vi "cursor window logic V2.vi"(4 "h. offset":dbl, 6 "CursIdx":i32, 7 "cursor window action":T2=enum."check", 8 "window":dbl=nan, 9 "center":dbl=nan, 10 "cursor window in":refnum<vi>, 11 "cursor window init":T1={"left"=2378.60310421286, "right "=2421.6740576496672, "center"=2421.6740576496672, "window"=2421.6740576496672, "cursors"=[], "relative"=0, "absolute"=0, "fixed vertical offset"=2421.6740576496672, "vertical offset"=2421.6740576496672, "skew"=2421.6740576496672, "default window frac"=2421.6740576496672, "kind"=enum."skewed", "skew.left"=2421.6740576496672, "skew.right"=2421.6740576496672, "Plot ref"=refnum, "wing order"=enum."back"}) -> (2 "cursor window out":refnum<vi>, 3 "cursor window out":T1={"left"=2378.60310421286, "right "=2421.6740576496672, "center"=2421.6740576496672, "window"=2421.6740576496672, "cursors"=[], "relative"=0, "absolute"=0, "fixed vertical offset"=2421.6740576496672, "vertical offset"=2421.6740576496672, "skew"=2421.6740576496672, "default window frac"=2421.6740576496672, "kind"=enum."skewed", "skew.left"=2421.6740576496672, "skew.right"=2421.6740576496672, "Plot ref"=refnum, "wing order"=enum."back"})   [LabVIEW 2015]
uses:
  cursor window action.ctl
  cursor winow.ctl
  stack action -- control.ctl
  Q - not nan -- real.vi
  Q - not nan -- integer.vi
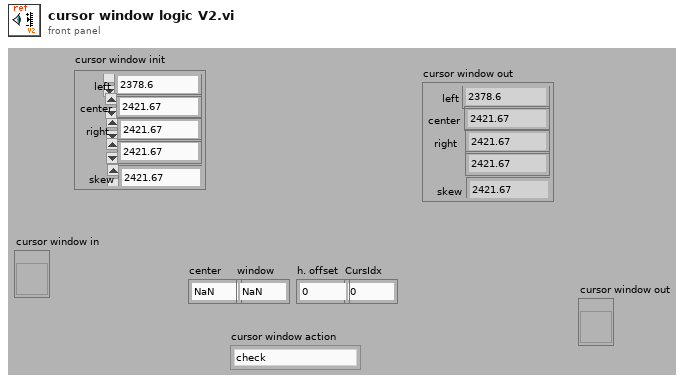
[diagram p1: front panel]
types:
  T1 = typedef "cursor winow.ctl" = cluster{"left":dbl, "right ":dbl, "center":dbl, "window":dbl, "cursors":i32[], "relative":i32, "absolute":i32, "fixed vertical offset":dbl, "vertical offset":dbl, "skew":dbl, "default window frac":dbl, "kind":enum16{"symmetric", "skewed", "fancy"}, "skew.left":dbl, "skew.right":dbl, "Plot ref":refnum<vi>, "wing order":enum16{"forw", "back"}}
  T2 = typedef "cursor window action.ctl" = enum16{"balance", "h. offset change", "cursor moves", "change center", "change window", "init", "check", "reset", "set y to middle", "idle", "-write all Y", "-write left.X", "-write center.X", "-write right.X", "-write all X", "-change center", "-change window", "-change skew", "-read cursor 2", "-read cursor 1", "-read cursor 0", "-read all cursors", "-reset", "-read plot scale", "-set y to middle", "-Q: center.Y is visible", "-Q: window is visible", "-parse center.Y", "-right left from center", "-left move", "-right move", "-set center.Y", "-empty", "-set cursors to default", "-check", "-write center.Y", "-copy cursor 1", "-copy cursor 0", "-copy cursor 2", "move right", "move left", "shrink", "broaden", "skew up", "skew down", "-write plot scale", "zoom X", "change cen&win", "zoom to all data"}
  T3 = typedef "stack action -- control.ctl" = enum16{"push", "pop", "check", "init"}
  T4 = cluster{"center":dbl, "window":dbl, "h.offset":dbl, "cursor window":T1}
  T5 = cluster{"right.Y":dbl, "right.X":dbl, "left.X":dbl, "left.Y":dbl, "center.X":dbl, "center.Y":dbl, "scale.x.max":dbl, "scale.x.min":dbl, "scale.y.range":dbl, "scale.y.min":dbl, "scale.x.range":dbl, "scale.y.max":dbl, "skew":dbl, "cursor":i32, "scale.x.center":dbl, "scale.x.halfwidth":dbl, "scale.y.center":dbl, "scale.y.halfwidth":dbl}
  T6 = cluster{"left":dbl, "right ":dbl, "center":dbl, "window":dbl, "cursors":i32[], "relative":i32, "absolute":i32, "fixed vertical offset":dbl, "vertical offset":dbl, "skew":dbl, "default window frac":dbl, "kind":enum16{"symmetric", "skewed", "fancy"}, "skew.left":dbl, "skew.right":dbl, "Plot ref":refnum<vi>, "wing order":enum16{"forw", "back"}}
  T7 = typedef "comparison control.ctl" = enum16{"not a number", "above", "in range", "below"}
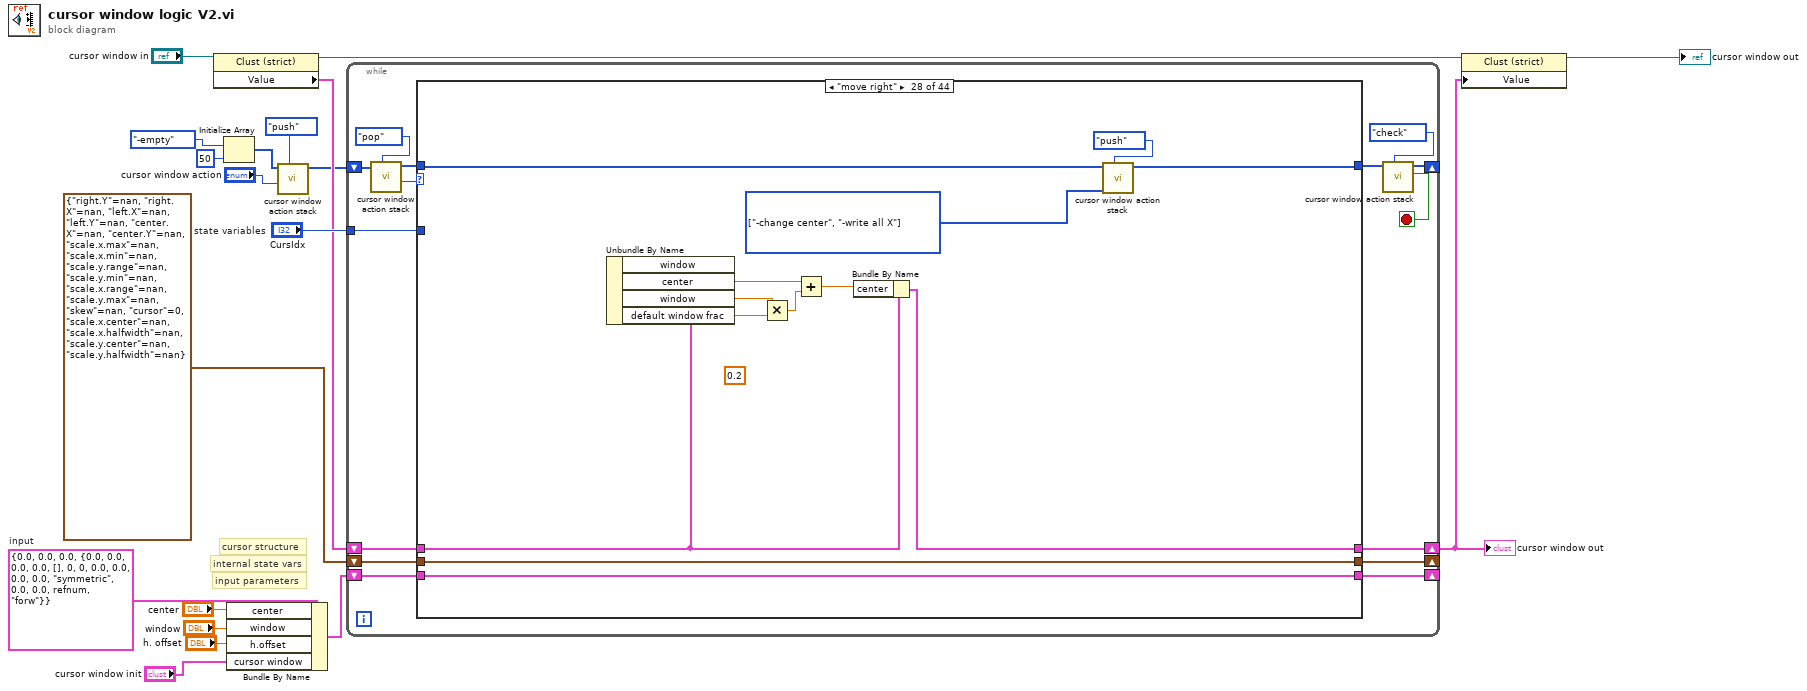
[diagram p0: block diagram]
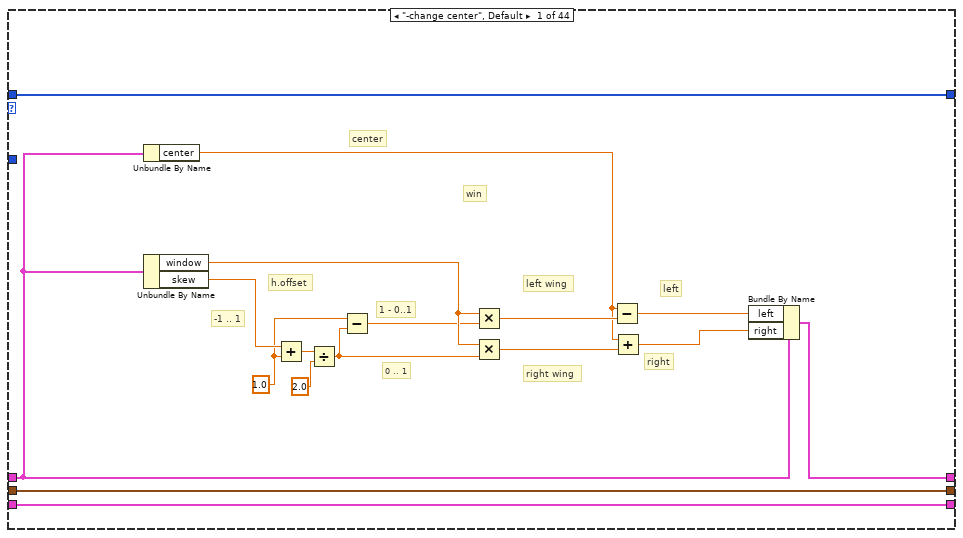
[diagram p2: hidden frame]
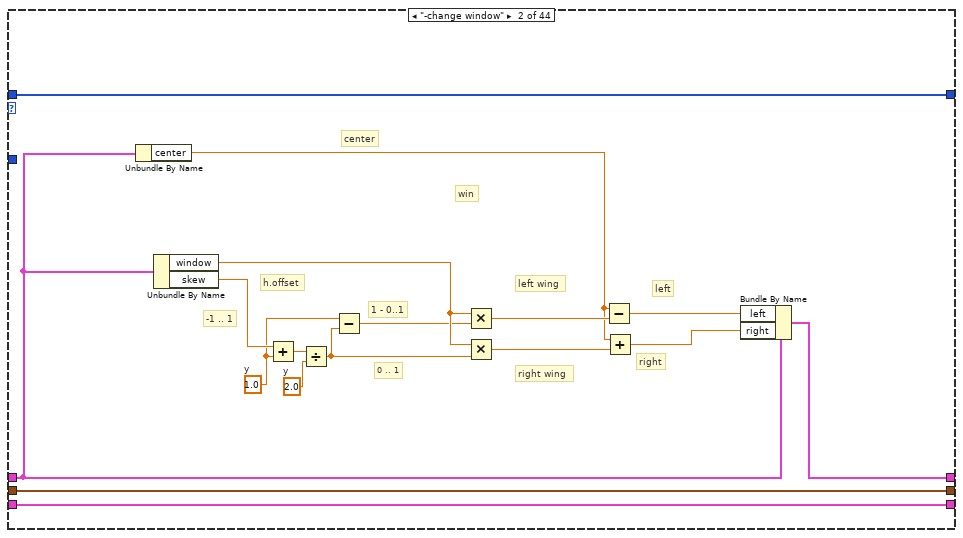
[diagram p3: hidden frame]
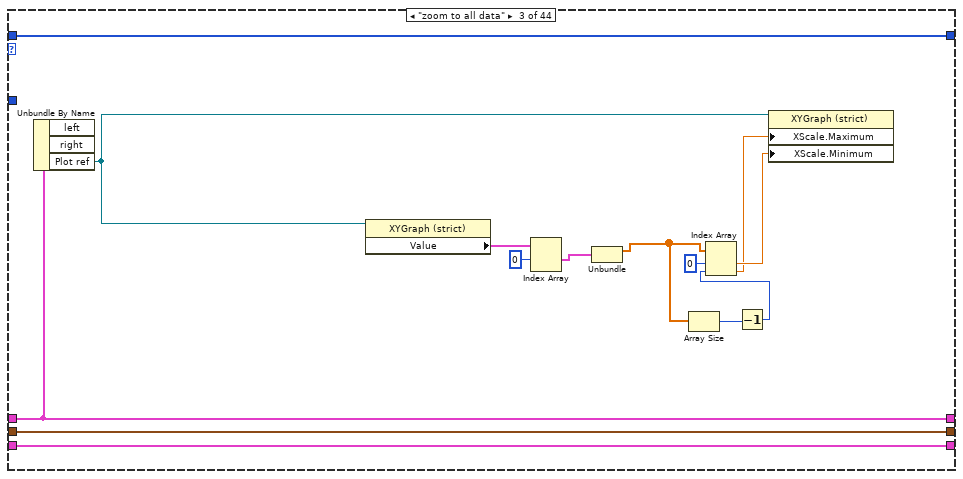
[diagram p4: hidden frame]
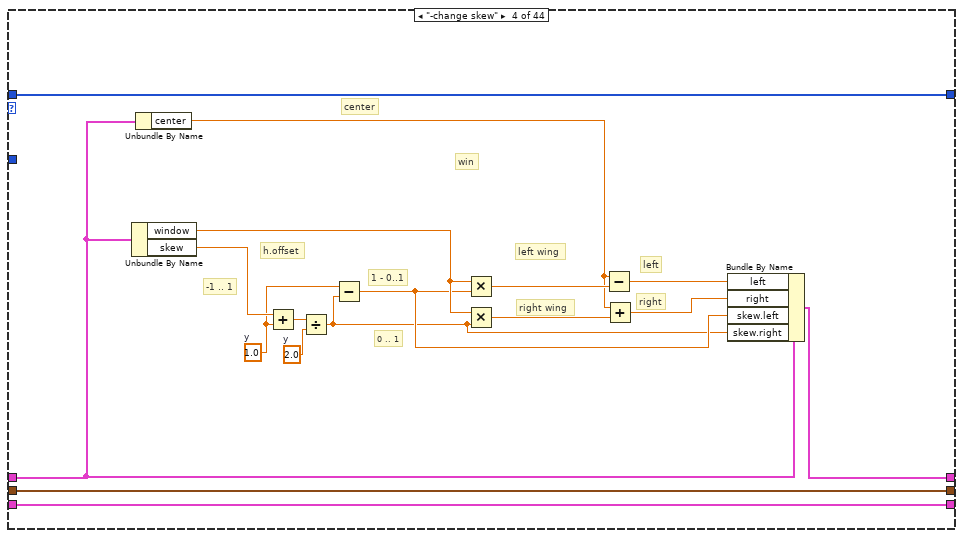
[diagram p5: hidden frame]
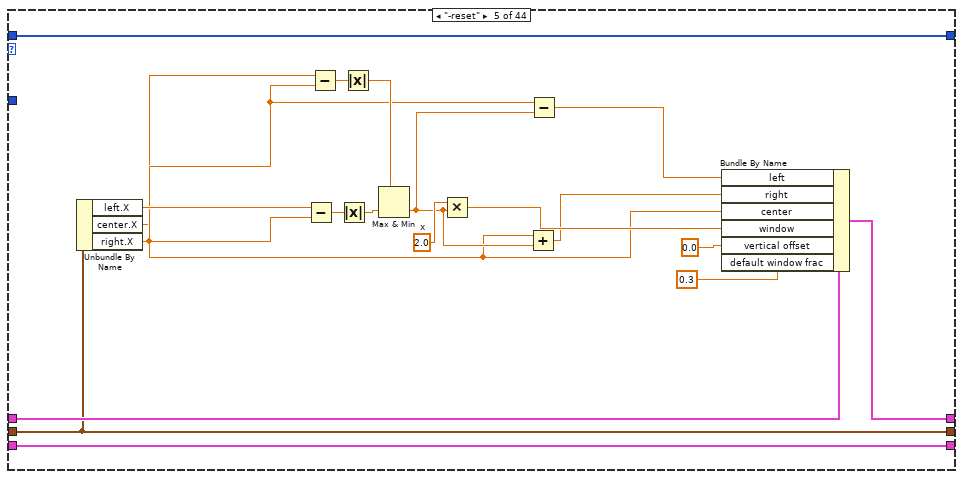
[diagram p6: hidden frame]
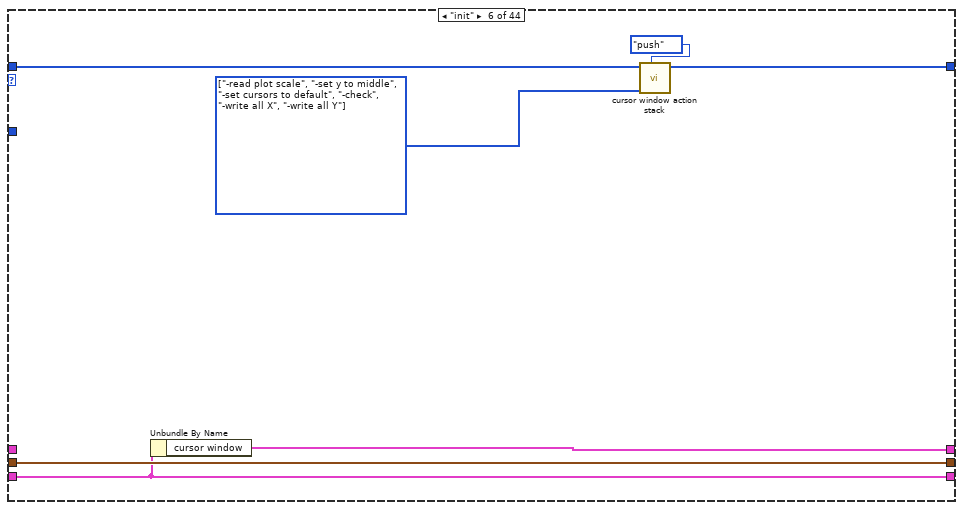
[diagram p7: hidden frame]
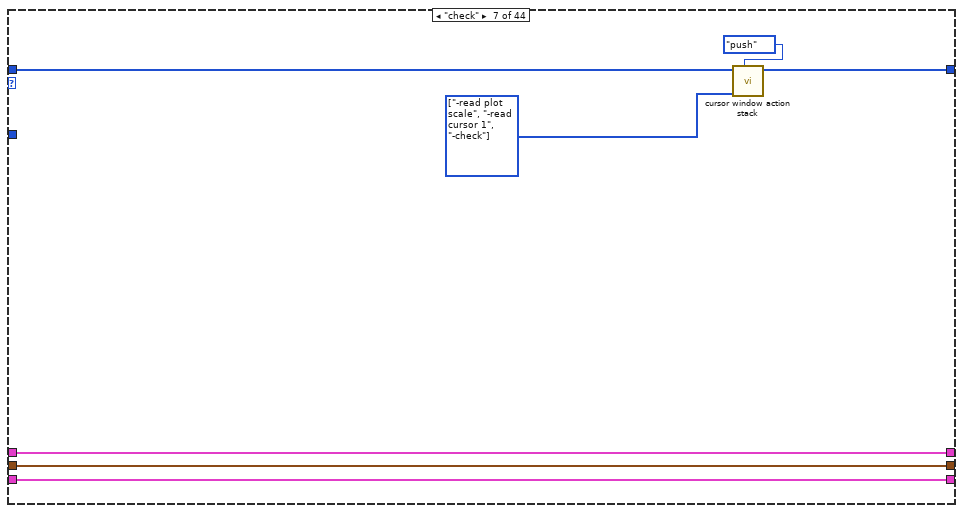
[diagram p8: hidden frame]
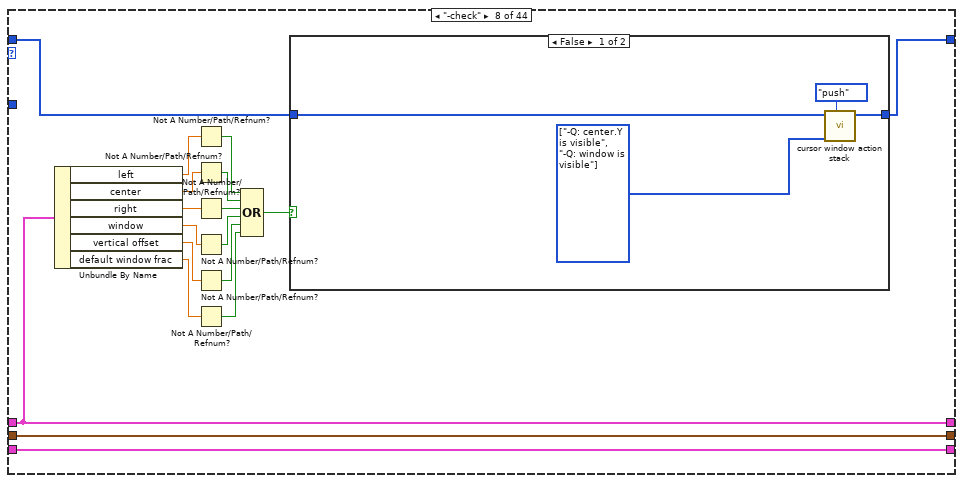
[diagram p9: hidden frame]
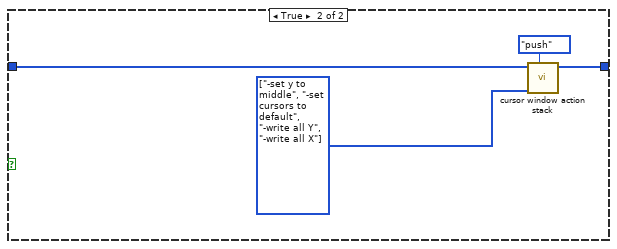
[diagram p10: hidden frame]
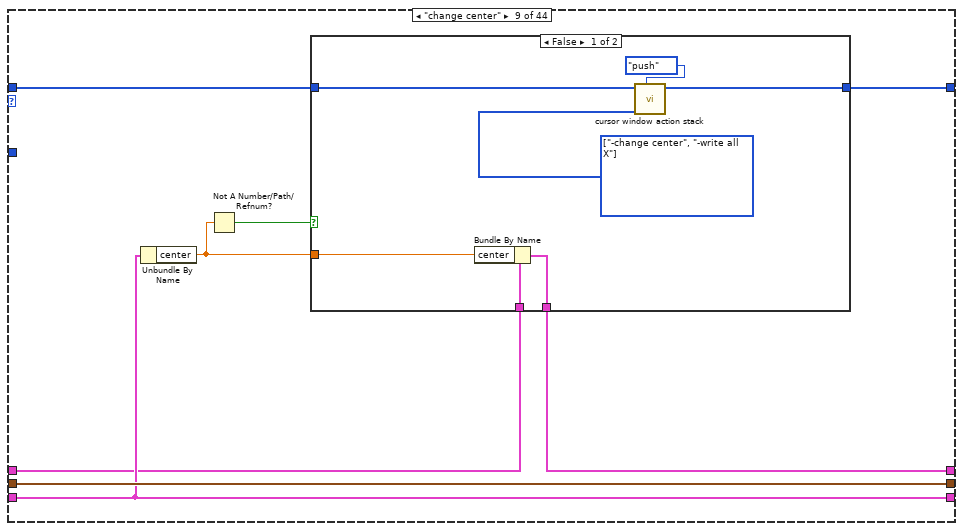
[diagram p11: hidden frame]
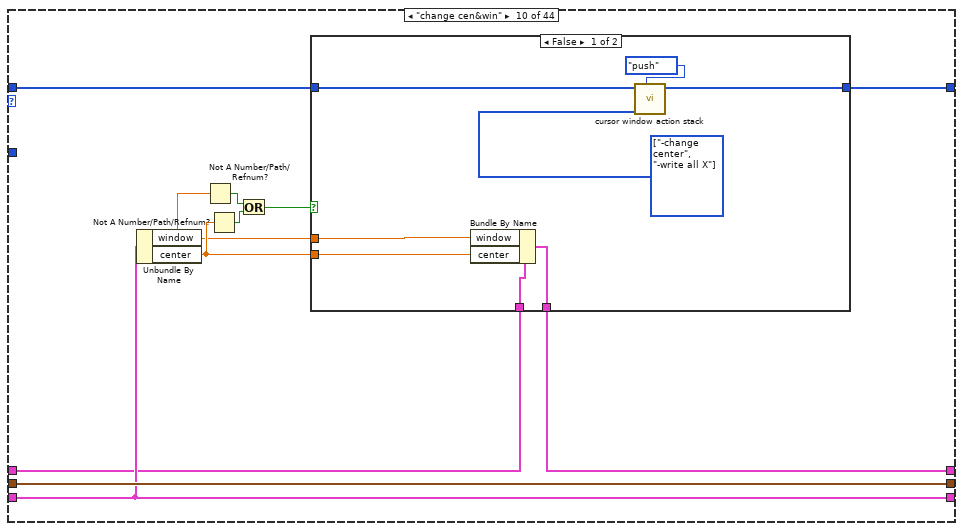
[diagram p13: hidden frame]
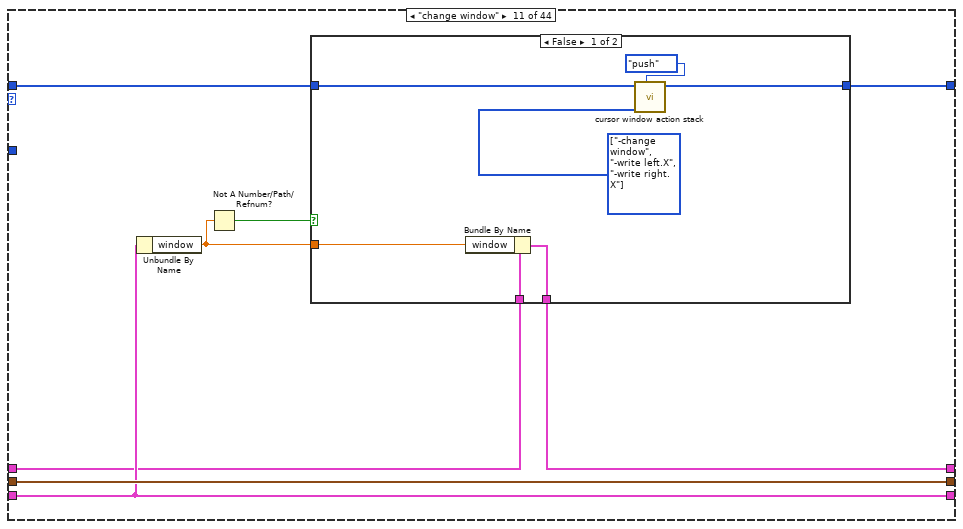
[diagram p15: hidden frame]
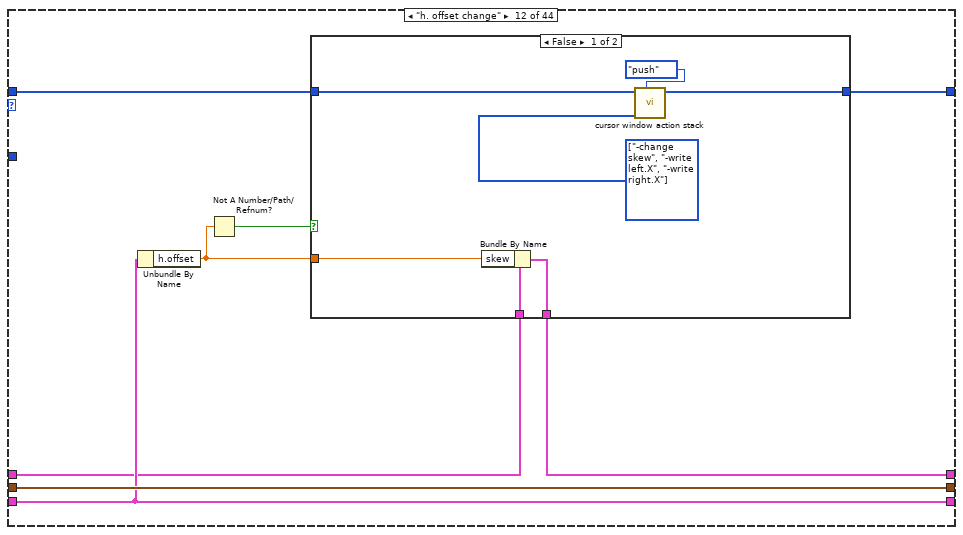
[diagram p17: hidden frame]
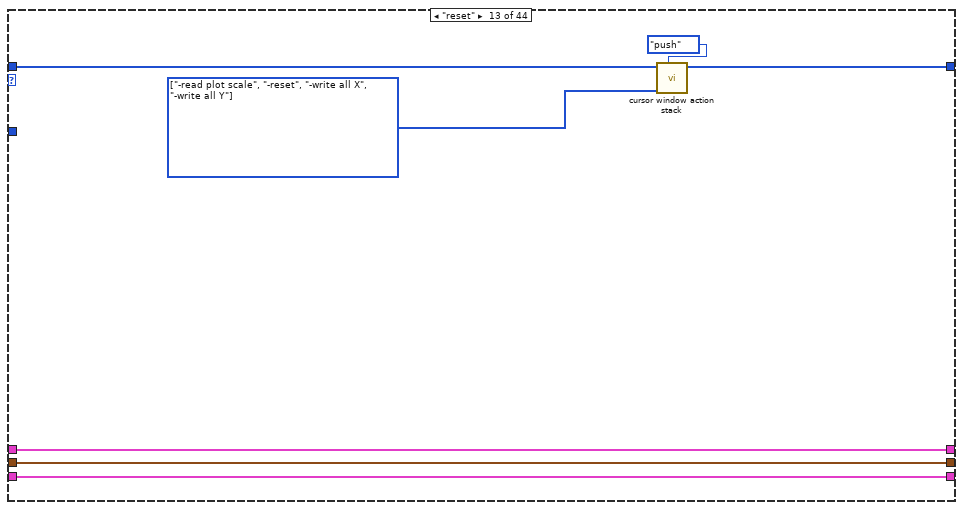
[diagram p19: hidden frame]
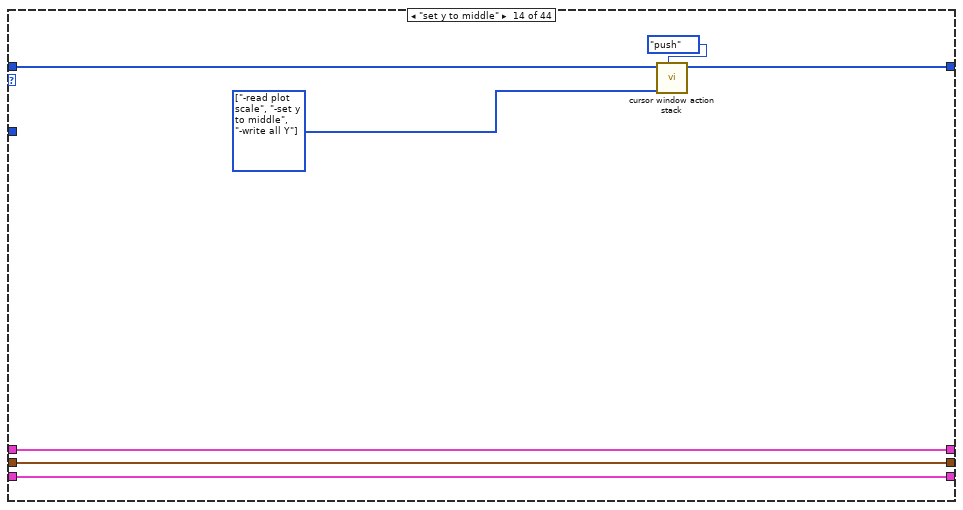
[diagram p20: hidden frame]
diagram:
  w17 = T4 {"center"=0.0, "window"=0.0, "h.offset"=0.0, "cursor window"={"left"=0.0, "right "=0.0, "center"=0.0, "window"=0.0, "cursors"=[], "relative"=0, "absolute"=0, "fixed vertical offset"=0.0, "vertical offset"=0.0, "skew"=0.0, "default window frac"=0.0, "kind"=enum."symmetric", "skew.left"=0.0, "skew.right"=0.0, "Plot ref"=refnum, "wing order"=enum."forw"}}  # input
  w18 = T5 {"right.Y"=nan, "right.X"=nan, "left.X"=nan, "left.Y"=nan, "center.X"=nan, "center.Y"=nan, "scale.x.max"=nan, "scale.x.min"=nan, "scale.y.range"=nan, "scale.y.min"=nan, "scale.x.range"=nan, "scale.y.max"=nan, "skew"=nan, "cursor"=0, "scale.x.center"=nan, "scale.x.halfwidth"=nan, "scale.y.center"=nan, "scale.y.halfwidth"=nan}  # state variables
  # "input parameters"
  # "internal state vars"
  # "cursor structure"
  n1 = property class="Clust (strict)"(reference="cursor window in") -> (reference out=w19:refnum<vi>, "Value"=w11:T6)  [unwired: 1 in, 1 out]
  n2 = Initialize Array(cursor_window_action."-empty" ("cursor window action"), 50 ("dimension size")) -> (w4:T2[])
  n3 = Bundle By Name(cluster=w17, "center"="center", "window"="window", "h.offset"="h. offset", "cursor window"="cursor window init") -> (w13:T4)
  n4 = call "cursor window action stack.vi"("stack action"=stack_action_--_control."push", "cursor window action"="cursor window action", "command stack"=w4) -> ("command stack out"=w3:T2[])  [unwired: 6 in, 2 out]
  n5 = while {
    shift-right: [w27] -> _
    shift-left: w3 -> [w33]
    shift-right: [w20] -> w10
    shift-left: w11 -> [w34]
    shift-right: [w24] -> _
    shift-left: w13 -> [w25]
    shift-right: [w22] -> _
    shift-left: w18 -> [w23]
    tunnel: "CursIdx" -> [w21]
    stop <- w26 stop-if-true
    n6 = call "cursor window action stack.vi"("stack action"=stack_action_--_control."pop", "command stack"=w33) -> ("cursor window action out"=w32:T2, "command stack out"=w30:T2[])  [unwired: 7 in, 1 out]
    n7 = case shown="\"move right\"" w32 {
      tunnel: w34 -> [w36 w53 w79 w86 w108 _ w126 w136 w160 w181 w198 w215 w231 w238 w255 w289 w324 w363 w395 w406 w413 w432 w439 w468 w481 w489 w513 w519 w539 w545 w558 w579 w618 w652 w692 w714 w728 w745 w764 w777 w786 w809 w822 w836]
      tunnel: [w40 w57 w82 w90 w107 w120 w129 w133 w165 w185 w203 w220 w234 w241 w252 w286 w326 w364 w396 w404 w422 w438 w455 w470 w483 w487 w514 w527 w540 w554 w562 w583 w616 w654 w709 w727 w742 w759 w773 w785 w807 w821 w835 w849] -> w28
      tunnel: w30 -> [w40 w57 w82 w90 w107 w121 w130 w134 w164 w184 w202 w219 w235 w242 w252 w286 w326 w351 w396 w404 w422 w438 w455 w470 w483 w488 w515 w528 w541 w555 w563 w584 w616 w655 w709 w727 w742 w759 w773 w785 w807 w821 w835 w849]
      tunnel: w25 -> [w37 w54 w80 w87 w106 w124 w127 w137 w163 w183 w201 w218 w237 w244 w254 w288 w325 w356 w393 w407 w421 w437 w458 w471 w484 w495 w509 w525 w535 w552 w559 w580 w634 w659 w694 w716 w734 w752 w766 w779 w788 w811 w825 w839]
      tunnel: [w37 w54 w80 w87 w106 w124 w127 w137 w163 w183 w201 w218 w237 w244 w254 w288 w325 w356 w393 w407 w421 w437 w458 w471 w484 w495 w509 w525 w535 w552 w559 w580 w634 w659 w694 w716 w734 w752 w766 w779 w788 w811 w825 w839] -> w24
      tunnel: w23 -> [w39 w56 w81 w89 w105 w125 w128 w138 w166 w186 w204 w221 w236 w243 w253 w287 w330 w357 w394 w409 w418 w436 w457 w462 w475 w491 w510 w526 w536 w553 w560 w581 w622 w658 w695 w713 w735 w753 w767 w776 w796 w815 w829 w843]
      tunnel: [w39 w56 w81 w89 w105 w125 w128 w138 w166 w186 w204 w221 w236 w243 w253 w287 w329 w357 w394 w409 w417 w436 w456 w462 w475 w490 w510 w526 w536 w553 w560 w581 w625 w658 w695 w713 w735 w753 w767 w776 w795 w814 w828 w842] -> w22
      tunnel: w21 -> [_ _ _ _ _ _ _ _ _ _ _ _ _ _ _ _ _ w354 _ _ _ _ _ _ _ _ _ _ _ _ _ _ _ _ _ _ _ _ _ _ _ _ _ _]
      tunnel: [w35 w52 w79 w85 w101 w119 w126 w136 w159 w180 w197 w214 w231 w238 w245 w279 w324 w355 w395 w405 w412 w428 w439 w468 w481 w489 w512 w518 w538 w544 w561 w582 w614 w651 w692 w714 w728 w745 w764 w777 w786 w809 w822 w836] -> w20
      frame "-change center", Default {
        w45 = 1.0 ("y")
        # "1 - 0..1"
        # "right"
        # "left"
        # "win"
        # "h.offset"
        # "center"
        # "left wing"
        # "right wing"
        # "0 .. 1"
        # "-1 .. 1"
        n8 = Unbundle By Name(w36) -> ("center"=w38:dbl)
        n9 = Unbundle By Name(w36) -> ("window"=w50:dbl, "skew"=w51:dbl)
        n10 = Add(x=w51, y=w45) -> (x+y=w46:dbl)
        n11 = Divide(x=w46, y=2.0) -> (x/y=w42:dbl)
        n12 = Subtract(x=w45, y=w42) -> (x-y=w41:dbl)
        n13 = Multiply(x=w50, y=w41) -> (x*y=w44:dbl)
        n14 = Multiply(x=w50, y=w42) -> (x*y=w43:dbl)
        n15 = Subtract(x=w38, y=w44) -> (x-y=w49:dbl)
        n16 = Add(x=w38, y=w43) -> (x+y=w48:dbl)
        n17 = Bundle By Name(cluster=w36, "left"=w49, "right"=w48) -> (w35:T1)
      }
      frame "-change window" {
        w62 = 1.0  # y
        w64 = 2.0  # y
        # "1 - 0..1"
        # "right"
        # "left"
        # "win"
        # "h.offset"
        # "center"
        # "left wing"
        # "right wing"
        # "0 .. 1"
        # "-1 .. 1"
        n18 = Unbundle By Name(w53) -> ("center"=w55:dbl)
        n19 = Unbundle By Name(w53) -> ("window"=w67:dbl, "skew"=w68:dbl)
        n20 = Add(x=w68, y=w62) -> (x+y=w63:dbl)
        n21 = Divide(x=w63, y=w64) -> (x/y=w59:dbl)
        n22 = Subtract(x=w62, y=w59) -> (x-y=w58:dbl)
        n23 = Multiply(x=w67, y=w58) -> (x*y=w61:dbl)
        n24 = Multiply(x=w67, y=w59) -> (x*y=w60:dbl)
        n25 = Subtract(x=w55, y=w61) -> (x-y=w66:dbl)
        n26 = Add(x=w55, y=w60) -> (x+y=w65:dbl)
        n27 = Bundle By Name(cluster=w53, "left"=w66, "right"=w65) -> (w52:T1)
      }
      frame "zoom to all data" {
        n28 = Unbundle By Name(w79) -> ("Plot ref"=w78:refnum<vi>)  [unwired: 2 out]
        n29 = property class="XYGraph (strict)"(reference=w78) -> ("Value"=w77:cluster{"all rows":dbl[], "all rows":dbl[]}[])  [unwired: 1 in, 2 out]
        n30 = Index Array(array=w77, index #1=0 ("index")) -> (element #1=w75:cluster{"all rows":dbl[], "all rows":dbl[]})  [unwired: 1 in, 1 out]
        n31 = Unbundle(w75) -> ("all rows"=w73:dbl[])  [unwired: 1 out]
        n32 = Array Size(array=w73) -> (size(s)=w72:i32)
        n33 = Decrement(x=w72) -> (x-1=w71:i32)
        n34 = Index Array(array=w73, index #1=0 ("index"), index #2=w71) -> (element #1=w70:dbl, element #2=w69:dbl)
        n35 = property class="XYGraph (strict)"(reference=w78, "XScale.Maximum"=w69, "XScale.Minimum"=w70) -> ()  [unwired: 1 in, 2 out]
      }
      frame "-change skew" {
        w93 = 1.0  # y
        w95 = 2.0  # y
        # "1 - 0..1"
        # "right"
        # "left"
        # "win"
        # "h.offset"
        # "center"
        # "left wing"
        # "right wing"
        # "0 .. 1"
        # "-1 .. 1"
        n36 = Unbundle By Name(w86) -> ("window"=w98:dbl, "skew"=w99:dbl)
        n37 = Unbundle By Name(w86) -> ("center"=w88:dbl)
        n38 = Add(x=w99, y=w93) -> (x+y=w94:dbl)
        n39 = Divide(x=w94, y=w95) -> (x/y=w83:dbl)
        n40 = Subtract(x=w93, y=w83) -> (x-y=w84:dbl)
        n41 = Multiply(x=w98, y=w84) -> (x*y=w92:dbl)
        n42 = Multiply(x=w98, y=w83) -> (x*y=w91:dbl)
        n43 = Subtract(x=w88, y=w92) -> (x-y=w97:dbl)
        n44 = Add(x=w88, y=w91) -> (x+y=w96:dbl)
        n45 = Bundle By Name(cluster=w86, "left"=w97, "right"=w96, "skew.left"=w84, "skew.right"=w83) -> (w85:T1)
      }
      frame "-reset" {
        w114 = 2.0  # x
        n46 = Unbundle By Name(w105) -> ("left.X"=w104:dbl, "center.X"=w102:dbl, "right.X"=w103:dbl)
        n47 = Subtract(x=w104, y=w103) -> (x-y=w117:dbl)
        n48 = Subtract(x=w102, y=w103) -> (x-y=w118:dbl)
        n49 = Absolute Value(x=w117) -> (abs(x)=w115:dbl)
        n50 = Absolute Value(x=w118) -> (abs(x)=w116:dbl)
        n51 = Max & Min(x=w116, y=w115) -> (min(x,y)=w112:dbl)  [unwired: 1 out]
        n52 = Multiply(x=w114, y=w112) -> (x*y=w113:dbl)
        n53 = Add(x=w103, y=w112) -> (x+y=w110:dbl)
        n54 = Subtract(x=w103, y=w112) -> (x-y=w111:dbl)
        n55 = Bundle By Name(cluster=w108, "left"=w111, "right"=w110, "center"=w103, "window"=w113, "vertical offset"=0.0, "default window frac"=0.3) -> (w101:T1)
      }
      frame "init" {
        w122 = T2[] [enum."-read plot scale", enum."-set y to middle", enum."-set cursors to default", enum."-check", enum."-write all X", enum."-write all Y"] items=["balance", "h. offset change", "cursor moves", "change center", "change window", "init", "check", "reset", "set y to middle", "idle", "-write all Y", "-write left.X", "-write center.X", "-write right.X", "-write all X", "-change center", "-change window", "-change skew", "-read cursor 2", "-read cursor 1", "-read cursor 0", "-read all cursors", "-reset", "-read plot scale", "-set y to middle", "-Q: center.Y is visible", "-Q: window is visible", "-parse center.Y", "-right left from center", "-left move", "-right move", "-set center.Y", "-empty", "-set cursors to default", "-check", "-write center.Y", "-copy cursor 1", "-copy cursor 0", "-copy cursor 2", "move right", "move left", "shrink", "broaden", "skew up", "skew down", "-write plot scale", "zoom X", "change cen&win", "zoom to all data"]
        n56 = Unbundle By Name(w124) -> ("cursor window"=w119:T1)
        n57 = call "cursor window action stack.vi"("stack action"=stack_action_--_control."push", "action list"=w122, "command stack"=w121) -> ("command stack out"=w120:T2[])  [unwired: 6 in, 2 out]
      }
      frame "check" {
        w131 = T2[] [enum."-read plot scale", enum."-read cursor 1", enum."-check"] items=["balance", "h. offset change", "cursor moves", "change center", "change window", "init", "check", "reset", "set y to middle", "idle", "-write all Y", "-write left.X", "-write center.X", "-write right.X", "-write all X", "-change center", "-change window", "-change skew", "-read cursor 2", "-read cursor 1", "-read cursor 0", "-read all cursors", "-reset", "-read plot scale", "-set y to middle", "-Q: center.Y is visible", "-Q: window is visible", "-parse center.Y", "-right left from center", "-left move", "-right move", "-set center.Y", "-empty", "-set cursors to default", "-check", "-write center.Y", "-copy cursor 1", "-copy cursor 0", "-copy cursor 2", "move right", "move left", "shrink", "broaden", "skew up", "skew down", "-write plot scale", "zoom X", "change cen&win", "zoom to all data"]
        n58 = call "cursor window action stack.vi"("stack action"=stack_action_--_control."push", "action list"=w131, "command stack"=w130) -> ("command stack out"=w129:T2[])  [unwired: 6 in, 2 out]
      }
      frame "-check" {
        n59 = Unbundle By Name(w136) -> ("left"=w148:dbl, "center"=w147:dbl, "right"=w149:dbl, "window"=w150:dbl, "vertical offset"=w142:dbl, "default window frac"=w141:dbl)
        n60 = Not A Number/Path/Refnum?(number/path/refnum=w148) -> (NaN/Path/Refnum?=w146:bool)
        n61 = Not A Number/Path/Refnum?(number/path/refnum=w147) -> (NaN/Path/Refnum?=w145:bool)
        n62 = Not A Number/Path/Refnum?(number/path/refnum=w149) -> (NaN/Path/Refnum?=w144:bool)
        n63 = Not A Number/Path/Refnum?(number/path/refnum=w150) -> (NaN/Path/Refnum?=w143:bool)
        n64 = Not A Number/Path/Refnum?(number/path/refnum=w142) -> (NaN/Path/Refnum?=w139:bool)
        n65 = Not A Number/Path/Refnum?(number/path/refnum=w141) -> (NaN/Path/Refnum?=w140:bool)
        n66 = Compound Arithmetic op=OR(w146, w145, w144, w143, w139, w140) -> (w135:bool)
        n67 = case shown="False" w135 {
          tunnel: w134 -> [w152 w156]
          tunnel: [w151 w155] -> w133
          frame False {
            w153 = T2[] [enum."-Q: center.Y is visible", enum."-Q: window is visible"] items=["balance", "h. offset change", "cursor moves", "change center", "change window", "init", "check", "reset", "set y to middle", "idle", "-write all Y", "-write left.X", "-write center.X", "-write right.X", "-write all X", "-change center", "-change window", "-change skew", "-read cursor 2", "-read cursor 1", "-read cursor 0", "-read all cursors", "-reset", "-read plot scale", "-set y to middle", "-Q: center.Y is visible", "-Q: window is visible", "-parse center.Y", "-right left from center", "-left move", "-right move", "-set center.Y", "-empty", "-set cursors to default", "-check", "-write center.Y", "-copy cursor 1", "-copy cursor 0", "-copy cursor 2", "move right", "move left", "shrink", "broaden", "skew up", "skew down", "-write plot scale", "zoom X", "change cen&win", "zoom to all data"]
            n68 = call "cursor window action stack.vi"("stack action"=stack_action_--_control."push", "action list"=w153, "command stack"=w152) -> ("command stack out"=w151:T2[])  [unwired: 6 in, 2 out]
          }
          frame True {
            w157 = T2[] [enum."-set y to middle", enum."-set cursors to default", enum."-write all Y", enum."-write all X"] items=["balance", "h. offset change", "cursor moves", "change center", "change window", "init", "check", "reset", "set y to middle", "idle", "-write all Y", "-write left.X", "-write center.X", "-write right.X", "-write all X", "-change center", "-change window", "-change skew", "-read cursor 2", "-read cursor 1", "-read cursor 0", "-read all cursors", "-reset", "-read plot scale", "-set y to middle", "-Q: center.Y is visible", "-Q: window is visible", "-parse center.Y", "-right left from center", "-left move", "-right move", "-set center.Y", "-empty", "-set cursors to default", "-check", "-write center.Y", "-copy cursor 1", "-copy cursor 0", "-copy cursor 2", "move right", "move left", "shrink", "broaden", "skew up", "skew down", "-write plot scale", "zoom X", "change cen&win", "zoom to all data"]
            n69 = call "cursor window action stack.vi"("stack action"=stack_action_--_control."push", "action list"=w157, "command stack"=w156) -> ("command stack out"=w155:T2[])  [unwired: 6 in, 2 out]
          }
        }
      }
      frame "change center" {
        n70 = Unbundle By Name(w163) -> ("center"=w161:dbl)
        n71 = Not A Number/Path/Refnum?(number/path/refnum=w161) -> (NaN/Path/Refnum?=w162:bool)
        n72 = case shown="False" w162 {
          tunnel: [w173 w174] -> w165
          tunnel: w164 -> [w172 w174]
          tunnel: w160 -> [w169 w175]
          tunnel: w161 -> [w168 _]
          tunnel: [w167 w175] -> w159
          frame False {
            w170 = T2[] [enum."-change center", enum."-write all X"] items=["balance", "h. offset change", "cursor moves", "change center", "change window", "init", "check", "reset", "set y to middle", "idle", "-write all Y", "-write left.X", "-write center.X", "-write right.X", "-write all X", "-change center", "-change window", "-change skew", "-read cursor 2", "-read cursor 1", "-read cursor 0", "-read all cursors", "-reset", "-read plot scale", "-set y to middle", "-Q: center.Y is visible", "-Q: window is visible", "-parse center.Y", "-right left from center", "-left move", "-right move", "-set center.Y", "-empty", "-set cursors to default", "-check", "-write center.Y", "-copy cursor 1", "-copy cursor 0", "-copy cursor 2", "move right", "move left", "shrink", "broaden", "skew up", "skew down", "-write plot scale", "zoom X", "change cen&win", "zoom to all data"]
            n73 = Bundle By Name(cluster=w169, "center"=w168) -> (w167:T1)
            n74 = call "cursor window action stack.vi"("stack action"=stack_action_--_control."push", "action list"=w170, "command stack"=w172) -> ("command stack out"=w173:T2[])  [unwired: 6 in, 2 out]
          }
          frame True {
          }
        }
      }
      frame "change cen&win" {
        n75 = Unbundle By Name(w183) -> ("window"=w176:dbl, "center"=w182:dbl)
        n76 = Not A Number/Path/Refnum?(number/path/refnum=w176) -> (NaN/Path/Refnum?=w179:bool)
        n77 = Not A Number/Path/Refnum?(number/path/refnum=w182) -> (NaN/Path/Refnum?=w178:bool)
        n78 = Or(x=w179, y=w178) -> (x .or. y?=w177:bool)
        n79 = case shown="False" w177 {
          tunnel: [w194 w195] -> w185
          tunnel: w184 -> [w193 w195]
          tunnel: w181 -> [w190 w196]
          tunnel: w182 -> [w189 _]
          tunnel: [w188 w196] -> w180
          tunnel: w176 -> [w187 _]
          frame False {
            w191 = T2[] [enum."-change center", enum."-write all X"] items=["balance", "h. offset change", "cursor moves", "change center", "change window", "init", "check", "reset", "set y to middle", "idle", "-write all Y", "-write left.X", "-write center.X", "-write right.X", "-write all X", "-change center", "-change window", "-change skew", "-read cursor 2", "-read cursor 1", "-read cursor 0", "-read all cursors", "-reset", "-read plot scale", "-set y to middle", "-Q: center.Y is visible", "-Q: window is visible", "-parse center.Y", "-right left from center", "-left move", "-right move", "-set center.Y", "-empty", "-set cursors to default", "-check", "-write center.Y", "-copy cursor 1", "-copy cursor 0", "-copy cursor 2", "move right", "move left", "shrink", "broaden", "skew up", "skew down", "-write plot scale", "zoom X", "change cen&win", "zoom to all data"]
            n80 = Bundle By Name(cluster=w190, "window"=w187, "center"=w189) -> (w188:T1)
            n81 = call "cursor window action stack.vi"("stack action"=stack_action_--_control."push", "action list"=w191, "command stack"=w193) -> ("command stack out"=w194:T2[])  [unwired: 6 in, 2 out]
          }
          frame True {
          }
        }
      }
      frame "change window" {
        n82 = Unbundle By Name(w201) -> ("window"=w199:dbl)
        n83 = Not A Number/Path/Refnum?(number/path/refnum=w199) -> (NaN/Path/Refnum?=w200:bool)
        n84 = case shown="False" w200 {
          tunnel: [w211 w212] -> w203
          tunnel: w202 -> [w210 w212]
          tunnel: w198 -> [w207 w213]
          tunnel: w199 -> [w206 _]
          tunnel: [w205 w213] -> w197
          frame False {
            w208 = T2[] [enum."-change window", enum."-write left.X", enum."-write right.X"] items=["balance", "h. offset change", "cursor moves", "change center", "change window", "init", "check", "reset", "set y to middle", "idle", "-write all Y", "-write left.X", "-write center.X", "-write right.X", "-write all X", "-change center", "-change window", "-change skew", "-read cursor 2", "-read cursor 1", "-read cursor 0", "-read all cursors", "-reset", "-read plot scale", "-set y to middle", "-Q: center.Y is visible", "-Q: window is visible", "-parse center.Y", "-right left from center", "-left move", "-right move", "-set center.Y", "-empty", "-set cursors to default", "-check", "-write center.Y", "-copy cursor 1", "-copy cursor 0", "-copy cursor 2", "move right", "move left", "shrink", "broaden", "skew up", "skew down", "-write plot scale", "zoom X", "change cen&win", "zoom to all data"]
            n85 = Bundle By Name(cluster=w207, "window"=w206) -> (w205:T1)
            n86 = call "cursor window action stack.vi"("stack action"=stack_action_--_control."push", "action list"=w208, "command stack"=w210) -> ("command stack out"=w211:T2[])  [unwired: 6 in, 2 out]
          }
          frame True {
          }
        }
      }
      frame "h. offset change" {
        n87 = Unbundle By Name(w218) -> ("h.offset"=w216:dbl)
        n88 = Not A Number/Path/Refnum?(number/path/refnum=w216) -> (NaN/Path/Refnum?=w217:bool)
        n89 = case shown="False" w217 {
          tunnel: [w228 w229] -> w220
          tunnel: w219 -> [w227 w229]
          tunnel: w215 -> [w224 w230]
          tunnel: w216 -> [w223 _]
          tunnel: [w222 w230] -> w214
          frame False {
            w225 = T2[] [enum."-change skew", enum."-write left.X", enum."-write right.X"] items=["balance", "h. offset change", "cursor moves", "change center", "change window", "init", "check", "reset", "set y to middle", "idle", "-write all Y", "-write left.X", "-write center.X", "-write right.X", "-write all X", "-change center", "-change window", "-change skew", "-read cursor 2", "-read cursor 1", "-read cursor 0", "-read all cursors", "-reset", "-read plot scale", "-set y to middle", "-Q: center.Y is visible", "-Q: window is visible", "-parse center.Y", "-right left from center", "-left move", "-right move", "-set center.Y", "-empty", "-set cursors to default", "-check", "-write center.Y", "-copy cursor 1", "-copy cursor 0", "-copy cursor 2", "move right", "move left", "shrink", "broaden", "skew up", "skew down", "-write plot scale", "zoom X", "change cen&win", "zoom to all data"]
            n90 = Bundle By Name(cluster=w224, "skew"=w223) -> (w222:T1)
            n91 = call "cursor window action stack.vi"("stack action"=stack_action_--_control."push", "action list"=w225, "command stack"=w227) -> ("command stack out"=w228:T2[])  [unwired: 6 in, 2 out]
          }
          frame True {
          }
        }
      }
      frame "reset" {
        w232 = T2[] [enum."-read plot scale", enum."-reset", enum."-write all X", enum."-write all Y"] items=["balance", "h. offset change", "cursor moves", "change center", "change window", "init", "check", "reset", "set y to middle", "idle", "-write all Y", "-write left.X", "-write center.X", "-write right.X", "-write all X", "-change center", "-change window", "-change skew", "-read cursor 2", "-read cursor 1", "-read cursor 0", "-read all cursors", "-reset", "-read plot scale", "-set y to middle", "-Q: center.Y is visible", "-Q: window is visible", "-parse center.Y", "-right left from center", "-left move", "-right move", "-set center.Y", "-empty", "-set cursors to default", "-check", "-write center.Y", "-copy cursor 1", "-copy cursor 0", "-copy cursor 2", "move right", "move left", "shrink", "broaden", "skew up", "skew down", "-write plot scale", "zoom X", "change cen&win", "zoom to all data"]
        n92 = call "cursor window action stack.vi"("stack action"=stack_action_--_control."push", "action list"=w232, "command stack"=w235) -> ("command stack out"=w234:T2[])  [unwired: 6 in, 2 out]
      }
      frame "set y to middle" {
        w239 = T2[] [enum."-read plot scale", enum."-set y to middle", enum."-write all Y"] items=["balance", "h. offset change", "cursor moves", "change center", "change window", "init", "check", "reset", "set y to middle", "idle", "-write all Y", "-write left.X", "-write center.X", "-write right.X", "-write all X", "-change center", "-change window", "-change skew", "-read cursor 2", "-read cursor 1", "-read cursor 0", "-read all cursors", "-reset", "-read plot scale", "-set y to middle", "-Q: center.Y is visible", "-Q: window is visible", "-parse center.Y", "-right left from center", "-left move", "-right move", "-set center.Y", "-empty", "-set cursors to default", "-check", "-write center.Y", "-copy cursor 1", "-copy cursor 0", "-copy cursor 2", "move right", "move left", "shrink", "broaden", "skew up", "skew down", "-write plot scale", "zoom X", "change cen&win", "zoom to all data"]
        n93 = call "cursor window action stack.vi"("stack action"=stack_action_--_control."push", "action list"=w239, "command stack"=w242) -> ("command stack out"=w241:T2[])  [unwired: 6 in, 2 out]
      }
      frame "-left move" {
        n94 = Unbundle By Name(w255) -> ("center"=w248:dbl, "skew.left"=w251:dbl, "skew.right"=w250:dbl)
        n95 = Unbundle By Name(w253) -> ("left.X"=w249:dbl)
        n96 = call "Q -- check range -- i -- real.vi"("upper"=w248, "number"=w249) -> ("selector"=w247:T7)  [unwired: 7 in, 2 out]
        n97 = case shown="\"in range\", Default" w247 {
          tunnel: w249 -> [w260 w278]
          tunnel: w250 -> [w266 w277]
          tunnel: [w267 w276] -> w256
          tunnel: [w262 w271] -> w258
          tunnel: w251 -> [w268 w275]
          tunnel: [w264 w270] -> w257
          tunnel: w248 -> [w261 w274]
          tunnel: [enum16{"forw", "back"}."forw" ("wing order") enum16{"forw", "back"}."back" ("wing order")] -> w246
          frame "in range", Default {
            # "right wing"
            # "left wing"
            n98 = Subtract(x=w261, y=w260) -> (x-y=w265:dbl)
            n99 = Divide(x=w265, y=w268) -> (x/y=w267:dbl)
            n100 = Multiply(x=w267, y=w266) -> (x*y=w263:dbl)
            n101 = Subtract(x=w261, y=w265) -> (x-y=w264:dbl)
            n102 = Add(x=w263, y=w261) -> (x+y=w262:dbl)
          }
          frame "above" {
            # "right wing"
            # "left wing"
            n103 = Subtract(x=w278, y=w274) -> (x-y=w273:dbl)
            n104 = Divide(x=w273, y=w277) -> (x/y=w276:dbl)
            n105 = Multiply(x=w276, y=w275) -> (x*y=w272:dbl)
            n106 = Subtract(x=w274, y=w272) -> (x-y=w270:dbl)
            n107 = Add(x=w273, y=w274) -> (x+y=w271:dbl)
          }
        }
        n108 = Bundle By Name(cluster=w255, "left"=w257, "right"=w258, "window"=w256, "wing order"=w246) -> (w245:T1)
      }
      frame "-right move" {
        n109 = Unbundle By Name(w289) -> ("center"=w280:dbl, "skew.left"=w285:dbl, "skew.right"=w284:dbl)
        n110 = Unbundle By Name(w287) -> ("right.X"=w283:dbl)
        n111 = call "Q -- check range -- i -- real.vi"("lower"=w280, "number"=w283) -> ("selector"=w282:T7)  [unwired: 7 in, 2 out]
        n112 = case shown="\"below\"" w282 {
          tunnel: w283 -> [w302 w304]
          tunnel: w284 -> [w301 w310]
          tunnel: [w300 w311] -> w290
          tunnel: [w295 w306] -> w292
          tunnel: w285 -> [w299 w312]
          tunnel: [w294 w308] -> w291
          tunnel: w280 -> [w298 w305]
          tunnel: [enum16{"forw", "back"}."forw" ("wing order") enum16{"forw", "back"}."back" ("wing order")] -> w281
          frame "in range", Default {
            # "right wing"
            n113 = Subtract(x=w302, y=w298) -> (x-y=w297:dbl)
            n114 = Divide(x=w297, y=w301) -> (x/y=w300:dbl)
            n115 = Multiply(x=w300, y=w299) -> (x*y=w296:dbl)
            n116 = Subtract(x=w298, y=w296) -> (x-y=w294:dbl)
            n117 = Add(x=w297, y=w298) -> (x+y=w295:dbl)
          }
          frame "below" {
            # "right wing"
            # "left wing"
            n118 = Subtract(x=w305, y=w304) -> (x-y=w309:dbl)
            n119 = Divide(x=w309, y=w312) -> (x/y=w311:dbl)
            n120 = Multiply(x=w311, y=w310) -> (x*y=w307:dbl)
            n121 = Subtract(x=w305, y=w309) -> (x-y=w308:dbl)
            n122 = Add(x=w307, y=w305) -> (x+y=w306:dbl)
          }
        }
        n123 = Bundle By Name(cluster=w289, "left"=w291, "right"=w292, "window"=w290, "wing order"=w281) -> (w279:T1)
      }
      frame "-set center.Y" {
        # "zero"
        # "calculate center.Y   from"
        # "complementary to calculation of fraction from vert offset"
        n124 = Unbundle By Name(w330) -> ("scale.y.halfwidth"=w327:dbl, "scale.y.center"=w328:dbl, "scale.x.range"=w334:dbl, "scale.y.max"=w333:dbl, "scale.y.min"=w332:dbl)
        n125 = Unbundle By Name(w324) -> ("window"=w335:dbl, "fixed vertical offset"=w336:dbl, "kind"=w314:enum16{"symmetric", "skewed", "fancy"}, "default window frac"=w337:dbl, "skew"=w313:dbl)
        n126 = case shown="\"symmetric\", Default" w314 {
          tunnel: w337 -> [w349 _]
          tunnel: w335 -> [w348 _]
          tunnel: w334 -> [w347 _]
          tunnel: [w338 w350] -> w315
          tunnel: w313 -> [_ w350]
          frame "symmetric", Default {
            # "window fraction"
            # "-1..1"
            n127 = Multiply(x=w347, y=w349) -> (x*y=w343:dbl)
            n128 = Divide(x=w348, y=w343) -> (x/y=w342:dbl)
            n129 = call "Q -- check range -- i -- real.vi"("upper"=0.99 ("y"), "lower"=0.0 ("y"), "number"=w342) -> ("number in range"=w339:dbl)  [unwired: 6 in, 2 out]
            n130 = Multiply(x=2.0, y=w339) -> (x*y=w346:dbl)
            n131 = Subtract(x=w346, y=1.0) -> (x-y=w338:dbl)
          }
          frame "skewed" {
          }
        }
        n132 = Multiply(x=w336, y=1.0) -> (x*y=w318:dbl)
        n133 = Multiply(x=w318, y=w327) -> (x*y=w323:dbl)
        n134 = Add(x=w328, y=w323) -> (x+y=w316:dbl)
        n135 = Subtract(x=w316, y=w332) -> (x-y=w321:dbl)
        n136 = Subtract(x=w333, y=w316) -> (x-y=w322:dbl)
        n137 = Max & Min(x=w322, y=w321) -> (min(x,y)=w320:dbl)  [unwired: 1 out]
        n138 = Multiply(x=w320, y=w315) -> (x*y=w317:dbl)
        n139 = Add(x=w316, y=w317) -> (x+y=w331:dbl)
        n140 = Bundle By Name(cluster=w330, "center.Y"=w331) -> (w329:T5)
      }
      frame "cursor moves" {
        n141 = Unbundle By Name(w363) -> ("cursors"=w362:i32[], "kind"=w353:enum16{"symmetric", "skewed", "fancy"})
        n142 = case shown="\"fancy\"" w353 {
          tunnel: [w365 w369] -> w352
          tunnel: w351 -> [w365 w368]
          frame "symmetric", Default {
          }
          frame "fancy" {
            n143 = call "cursor window action stack.vi"("stack action"=stack_action_--_control."push", "cursor window action"=cursor_window_action."-write plot scale", "command stack"=w368) -> ("command stack out"=w369:T2[])  [unwired: 6 in, 2 out]
          }
        }
        n144 = Array Max & Min(array=w362) -> (max value=w360:i32, min value=w359:i32)  [unwired: 2 out]
        n145 = call "Q -- check range -- i -- integer.vi"("upper"=w360, "lower"=w359, "number"=w354) -> ("in range?"=w358:bool)  [unwired: 6 in, 2 out]
        n146 = Subtract(x=w354, y=w359) -> (x-y=w361:i32)
        n147 = case shown="True" w358 {
          tunnel: w352 -> [w371 w378]
          tunnel: [w371 w377] -> w364
          tunnel: w363 -> [w370 w376]
          tunnel: [w370 w375] -> w355
          tunnel: w362 -> [_ w374]
          tunnel: w361 -> [_ w373]
          frame False {
          }
          frame True {
            n148 = Index Array(array=w374, index=w373) -> (element=w372:i32)
            n149 = Bundle By Name(cluster=w376, "absolute"=w372, "relative"=w373) -> (w375:T1)
            n150 = case shown="0, 2, Default" w373 {
              selector: w373 -> [_ w388]
              tunnel: w378 -> [w382 w390]
              tunnel: [w381 w389] -> w377
              frame 1 {
                w379 = T2[] [enum."-read cursor 1", enum."-read plot scale", enum."-parse center.Y", enum."-copy cursor 1", enum."-change center", enum."-write right.X", enum."-write left.X"] items=["balance", "h. offset change", "cursor moves", "change center", "change window", "init", "check", "reset", "set y to middle", "idle", "-write all Y", "-write left.X", "-write center.X", "-write right.X", "-write all X", "-change center", "-change window", "-change skew", "-read cursor 2", "-read cursor 1", "-read cursor 0", "-read all cursors", "-reset", "-read plot scale", "-set y to middle", "-Q: center.Y is visible", "-Q: window is visible", "-parse center.Y", "-right left from center", "-left move", "-right move", "-set center.Y", "-empty", "-set cursors to default", "-check", "-write center.Y", "-copy cursor 1", "-copy cursor 0", "-copy cursor 2", "move right", "move left", "shrink", "broaden", "skew up", "skew down", "-write plot scale", "zoom X", "change cen&win", "zoom to all data"]
                n151 = call "cursor window action stack.vi"("stack action"=stack_action_--_control."push", "action list"=w379, "command stack"=w382) -> ("command stack out"=w381:T2[])  [unwired: 6 in, 2 out]
              }
              frame 0, 2, Default {
                w387 = T2[] [enum."-set center.Y", enum."-write center.Y"] items=["balance", "h. offset change", "cursor moves", "change center", "change window", "init", "check", "reset", "set y to middle", "idle", "-write all Y", "-write left.X", "-write center.X", "-write right.X", "-write all X", "-change center", "-change window", "-change skew", "-read cursor 2", "-read cursor 1", "-read cursor 0", "-read all cursors", "-reset", "-read plot scale", "-set y to middle", "-Q: center.Y is visible", "-Q: window is visible", "-parse center.Y", "-right left from center", "-left move", "-right move", "-set center.Y", "-empty", "-set cursors to default", "-check", "-write center.Y", "-copy cursor 1", "-copy cursor 0", "-copy cursor 2", "move right", "move left", "shrink", "broaden", "skew up", "skew down", "-write plot scale", "zoom X", "change cen&win", "zoom to all data"]
                w385 = T2[] [enum."-read plot scale"] items=["balance", "h. offset change", "cursor moves", "change center", "change window", "init", "check", "reset", "set y to middle", "idle", "-write all Y", "-write left.X", "-write center.X", "-write right.X", "-write all X", "-change center", "-change window", "-change skew", "-read cursor 2", "-read cursor 1", "-read cursor 0", "-read all cursors", "-reset", "-read plot scale", "-set y to middle", "-Q: center.Y is visible", "-Q: window is visible", "-parse center.Y", "-right left from center", "-left move", "-right move", "-set center.Y", "-empty", "-set cursors to default", "-check", "-write center.Y", "-copy cursor 1", "-copy cursor 0", "-copy cursor 2", "move right", "move left", "shrink", "broaden", "skew up", "skew down", "-write plot scale", "zoom X", "change cen&win", "zoom to all data"]
                n152 = case shown="0, Default" w388 {
                  tunnel: [w391 w392] -> w386
                  frame 0, Default {
                    w391 = T2[] [enum."-read cursor 0", enum."-left move", enum."-write right.X"] items=["balance", "h. offset change", "cursor moves", "change center", "change window", "init", "check", "reset", "set y to middle", "idle", "-write all Y", "-write left.X", "-write center.X", "-write right.X", "-write all X", "-change center", "-change window", "-change skew", "-read cursor 2", "-read cursor 1", "-read cursor 0", "-read all cursors", "-reset", "-read plot scale", "-set y to middle", "-Q: center.Y is visible", "-Q: window is visible", "-parse center.Y", "-right left from center", "-left move", "-right move", "-set center.Y", "-empty", "-set cursors to default", "-check", "-write center.Y", "-copy cursor 1", "-copy cursor 0", "-copy cursor 2", "move right", "move left", "shrink", "broaden", "skew up", "skew down", "-write plot scale", "zoom X", "change cen&win", "zoom to all data"]
                  }
                  frame 2 {
                    w392 = T2[] [enum."-read cursor 2", enum."-right move", enum."-write left.X"] items=["balance", "h. offset change", "cursor moves", "change center", "change window", "init", "check", "reset", "set y to middle", "idle", "-write all Y", "-write left.X", "-write center.X", "-write right.X", "-write all X", "-change center", "-change window", "-change skew", "-read cursor 2", "-read cursor 1", "-read cursor 0", "-read all cursors", "-reset", "-read plot scale", "-set y to middle", "-Q: center.Y is visible", "-Q: window is visible", "-parse center.Y", "-right left from center", "-left move", "-right move", "-set center.Y", "-empty", "-set cursors to default", "-check", "-write center.Y", "-copy cursor 1", "-copy cursor 0", "-copy cursor 2", "move right", "move left", "shrink", "broaden", "skew up", "skew down", "-write plot scale", "zoom X", "change cen&win", "zoom to all data"]
                  }
                }
                n153 = Build Array (concatenate)(w385, w386, w387) -> (w383:T2[])
                n154 = call "cursor window action stack.vi"("stack action"=stack_action_--_control."push", "action list"=w383, "command stack"=w390) -> ("command stack out"=w389:T2[])  [unwired: 6 in, 2 out]
              }
            }
          }
        }
      }
      frame "idle" {
        n155 = disable-structure shown="Disabled" {
          frame Disabled {
            w397 = "win:left"  # Name
            w403 = u32 0  # Cursor Mode
            w402 = TRUE  # Allow Drag
            w401 = FALSE  # Name Visible
            w400 = u8 0  # Point Style
            w399 = u8 2  # Style
            n156 = Bundle By Name("Name"=w397, "Color"=u32 16768256, "Style"=w399, "Point Style"=w400, "Name Visible"=w401, "Allow Drag"=w402, "Cursor Mode"=w403) -> ()  [unwired: 1 in, 1 out]
            n157 = call "Q -- check range -- i -- real.vi"() -> ()  [unwired: 9 in, 3 out]
          }
          frame Enabled {
          }
        }
      }
      frame "-copy cursor 1" {
        n158 = Unbundle By Name(w409) -> ("center.X"=w408:dbl)
        n159 = Bundle By Name(cluster=w406, "center"=w408) -> (w405:T1)
      }
      frame "-set y to middle" {
        w410 = 0.5
        n160 = Unbundle By Name(w413) -> ("fixed vertical offset"=w419:dbl)
        n161 = Unbundle By Name(w418) -> ("scale.y.center"=w414:dbl, "scale.y.halfwidth"=w415:dbl)
        n162 = Multiply(x=w415, y=w419) -> (x*y=w420:dbl)
        n163 = Bundle By Name(cluster=w413, "skew"=0.0, "skew.left"=w410, "skew.right"=w410) -> (w412:T1)
        n164 = Add(x=w414, y=w420) -> (x+y=w416:dbl)
        n165 = Bundle By Name(cluster=w418, "right.Y"=w416, "center.Y"=w416, "left.Y"=w416) -> (w417:T5)
      }
      frame "-set cursors to default" {
        w426 = 0.5
        w425 = 0.1
        (unwired) 3
        n166 = Unbundle By Name(w436) -> ("scale.x.halfwidth"=w424:dbl, "scale.x.center"=w430:dbl)
        n167 = Multiply(x=w424, y=w425) -> (x*y=w423:dbl)
        n168 = Multiply(x=w423, y=2) -> (x*y=w429:dbl)
        n169 = Add(x=w430, y=w423) -> (x+y=w434:dbl)
        n170 = Subtract(x=w430, y=w423) -> (x-y=w435:dbl)
        n171 = Bundle By Name(cluster=w432, "vertical offset"=0.0, "default window frac"=w425, "left"=w435, "right"=w434, "center"=w430, "window"=w429, "skew"=0.0, "skew.left"=w426, "skew.right"=w426) -> (w428:T1)
      }
      frame "-read plot scale" {
        w446 = 2.0 ("y")
        w453 = 2.0 ("y")
        n172 = Unbundle By Name(w439) -> ("Plot ref"=w440:refnum<vi>)
        n173 = property on="Property Node" class="XYGraph (strict)"(reference=w440) -> ("YScale.Maximum"=w444:dbl, "YScale.Minimum"=w445:dbl, "XScale.Maximum"=w451:dbl, "XScale.Minimum"=w452:dbl)  [unwired: 1 in, 2 out]
        n174 = Add(x=w451, y=w452) -> (x+y=w454:dbl)
        n175 = Subtract(x=w451, y=w452) -> (x-y=w450:dbl)
        n176 = Divide(x=w454, y=w453) -> (x/y=w449:dbl)
        n177 = Divide(x=w450, y=w453) -> (x/y=w448:dbl)
        n178 = Subtract(x=w444, y=w445) -> (x-y=w441:dbl)
        n179 = Add(x=w444, y=w445) -> (x+y=w447:dbl)
        n180 = Divide(x=w447, y=w446) -> (x/y=w443:dbl)
        n181 = Divide(x=w441, y=w446) -> (x/y=w442:dbl)
        n182 = Bundle By Name(cluster=w457, "scale.y.max"=w444, "scale.y.min"=w445, "scale.x.max"=w451, "scale.x.min"=w452, "scale.x.range"=w450, "scale.x.halfwidth"=w448, "scale.x.center"=w449, "scale.y.range"=w441, "scale.y.halfwidth"=w442, "scale.y.center"=w443) -> (w456:T5)
      }
      frame "-write plot scale" {
        n183 = Unbundle By Name(w468) -> ("Plot ref"=w469:refnum<vi>, "window"=w467:dbl, "center"=w464:dbl, "default window frac"=w466:dbl)
        n184 = Divide(x=w467, y=w466) -> (x/y=w461:dbl)
        n185 = Divide(x=w461, y=2) -> (x/y=w460:dbl)
        n186 = Add(x=w464, y=w460) -> (x+y=w463:dbl)
        n187 = Subtract(x=w464, y=w460) -> (x-y=w465:dbl)
        n188 = property on="Property Node" class="XYGraph (strict)"(reference=w469, "XScale.Maximum"=w463, "XScale.Minimum"=w465) -> ()  [unwired: 1 in, 2 out]
      }
      frame "zoom X" {
        n189 = Unbundle By Name(w481) -> ("Plot ref"=w482:refnum<vi>, "window"=w480:dbl, "center"=w477:dbl, "default window frac"=w479:dbl)
        n190 = Divide(x=w480, y=w479) -> (x/y=w474:dbl)
        n191 = Divide(x=w474, y=1) -> (x/y=w473:dbl)
        n192 = Add(x=w477, y=w473) -> (x+y=w476:dbl)
        n193 = Subtract(x=w477, y=w473) -> (x-y=w478:dbl)
        n194 = property on="Property Node" class="XYGraph (strict)"(reference=w482, "XScale.Maximum"=w476, "XScale.Minimum"=w478) -> ()  [unwired: 1 in, 2 out]
      }
      frame "-Q: center.Y is visible" {
        # "check if y is within y-scale bounds"
        n195 = Unbundle By Name(w491) -> ("center.Y"=w494:dbl, "scale.y.max"=w493:dbl, "scale.y.min"=w492:dbl, "scale.y.center"=w485:dbl)
        n196 = call "Q -- check range -- i -- real.vi"("upper"=w493, "lower"=w492, "number"=w494) -> ("in range?"=w486:bool)  [unwired: 6 in, 2 out]
        n197 = case shown="False" w486 {
          tunnel: w491 -> [w502 w504]
          tunnel: [w501 w504] -> w490
          tunnel: w488 -> [w499 w503]
          tunnel: [w497 w503] -> w487
          tunnel: w485 -> [w496 _]
          frame False {
            w500 = T2[] [enum."-parse center.Y", enum."-write center.Y"] items=["balance", "h. offset change", "cursor moves", "change center", "change window", "init", "check", "reset", "set y to middle", "idle", "-write all Y", "-write left.X", "-write center.X", "-write right.X", "-write all X", "-change center", "-change window", "-change skew", "-read cursor 2", "-read cursor 1", "-read cursor 0", "-read all cursors", "-reset", "-read plot scale", "-set y to middle", "-Q: center.Y is visible", "-Q: window is visible", "-parse center.Y", "-right left from center", "-left move", "-right move", "-set center.Y", "-empty", "-set cursors to default", "-check", "-write center.Y", "-copy cursor 1", "-copy cursor 0", "-copy cursor 2", "move right", "move left", "shrink", "broaden", "skew up", "skew down", "-write plot scale", "zoom X", "change cen&win", "zoom to all data"]
            n198 = Bundle By Name(cluster=w502, "center.Y"=w496) -> (w501:T5)
            n199 = call "cursor window action stack.vi"("stack action"=stack_action_--_control."push", "action list"=w500, "command stack"=w499) -> ("command stack out"=w497:T2[])  [unwired: 6 in, 2 out]
          }
          frame True {
          }
        }
      }
      frame "move left" {
        (unwired) 0.2
        w517 = T2[] [enum."-change center", enum."-write all X"] items=["balance", "h. offset change", "cursor moves", "change center", "change window", "init", "check", "reset", "set y to middle", "idle", "-write all Y", "-write left.X", "-write center.X", "-write right.X", "-write all X", "-change center", "-change window", "-change skew", "-read cursor 2", "-read cursor 1", "-read cursor 0", "-read all cursors", "-reset", "-read plot scale", "-set y to middle", "-Q: center.Y is visible", "-Q: window is visible", "-parse center.Y", "-right left from center", "-left move", "-right move", "-set center.Y", "-empty", "-set cursors to default", "-check", "-write center.Y", "-copy cursor 1", "-copy cursor 0", "-copy cursor 2", "move right", "move left", "shrink", "broaden", "skew up", "skew down", "-write plot scale", "zoom X", "change cen&win", "zoom to all data"]
        n200 = Unbundle By Name(w513) -> ("center"=w507:dbl, "window"=w506:dbl, "default window frac"=w505:dbl)  [unwired: 1 out]
        n201 = Multiply(x=w506, y=w505) -> (x*y=w508:dbl)
        n202 = Subtract(x=w507, y=w508) -> (x-y=w511:dbl)
        n203 = Bundle By Name(cluster=w513, "center"=w511) -> (w512:T1)
        n204 = call "cursor window action stack.vi"("stack action"=stack_action_--_control."push", "action list"=w517, "command stack"=w515) -> ("command stack out"=w514:T2[])  [unwired: 6 in, 2 out]
      }
      frame "move right" {
        (unwired) 0.2
        w530 = T2[] [enum."-change center", enum."-write all X"] items=["balance", "h. offset change", "cursor moves", "change center", "change window", "init", "check", "reset", "set y to middle", "idle", "-write all Y", "-write left.X", "-write center.X", "-write right.X", "-write all X", "-change center", "-change window", "-change skew", "-read cursor 2", "-read cursor 1", "-read cursor 0", "-read all cursors", "-reset", "-read plot scale", "-set y to middle", "-Q: center.Y is visible", "-Q: window is visible", "-parse center.Y", "-right left from center", "-left move", "-right move", "-set center.Y", "-empty", "-set cursors to default", "-check", "-write center.Y", "-copy cursor 1", "-copy cursor 0", "-copy cursor 2", "move right", "move left", "shrink", "broaden", "skew up", "skew down", "-write plot scale", "zoom X", "change cen&win", "zoom to all data"]
        n205 = Unbundle By Name(w519) -> ("center"=w522:dbl, "window"=w521:dbl, "default window frac"=w520:dbl)  [unwired: 1 out]
        n206 = Multiply(x=w521, y=w520) -> (x*y=w523:dbl)
        n207 = Add(x=w522, y=w523) -> (x+y=w524:dbl)
        n208 = Bundle By Name(cluster=w519, "center"=w524) -> (w518:T1)
        n209 = call "cursor window action stack.vi"("stack action"=stack_action_--_control."push", "action list"=w530, "command stack"=w528) -> ("command stack out"=w527:T2[])  [unwired: 6 in, 2 out]
      }
      frame "shrink" {
        (unwired) 0.3
        w543 = T2[] [enum."-change window", enum."-write all X", enum."-read plot scale", enum."-set center.Y", enum."-write center.Y"] items=["balance", "h. offset change", "cursor moves", "change center", "change window", "init", "check", "reset", "set y to middle", "idle", "-write all Y", "-write left.X", "-write center.X", "-write right.X", "-write all X", "-change center", "-change window", "-change skew", "-read cursor 2", "-read cursor 1", "-read cursor 0", "-read all cursors", "-reset", "-read plot scale", "-set y to middle", "-Q: center.Y is visible", "-Q: window is visible", "-parse center.Y", "-right left from center", "-left move", "-right move", "-set center.Y", "-empty", "-set cursors to default", "-check", "-write center.Y", "-copy cursor 1", "-copy cursor 0", "-copy cursor 2", "move right", "move left", "shrink", "broaden", "skew up", "skew down", "-write plot scale", "zoom X", "change cen&win", "zoom to all data"]
        n210 = Unbundle By Name(w539) -> ("window"=w534:dbl, "window"=w533:dbl, "default window frac"=w531:dbl)
        n211 = Multiply(x=w533, y=w531) -> (x*y=w532:dbl)
        n212 = Subtract(x=w534, y=w532) -> (x-y=w537:dbl)
        n213 = Bundle By Name(cluster=w539, "window"=w537) -> (w538:T1)
        n214 = call "cursor window action stack.vi"("stack action"=stack_action_--_control."push", "action list"=w543, "command stack"=w541) -> ("command stack out"=w540:T2[])  [unwired: 6 in, 2 out]
      }
      frame "broaden" {
        (unwired) 0.3
        w551 = T2[] [enum."-change window", enum."-write all X", enum."-read plot scale", enum."-set center.Y", enum."-write center.Y"] items=["balance", "h. offset change", "cursor moves", "change center", "change window", "init", "check", "reset", "set y to middle", "idle", "-write all Y", "-write left.X", "-write center.X", "-write right.X", "-write all X", "-change center", "-change window", "-change skew", "-read cursor 2", "-read cursor 1", "-read cursor 0", "-read all cursors", "-reset", "-read plot scale", "-set y to middle", "-Q: center.Y is visible", "-Q: window is visible", "-parse center.Y", "-right left from center", "-left move", "-right move", "-set center.Y", "-empty", "-set cursors to default", "-check", "-write center.Y", "-copy cursor 1", "-copy cursor 0", "-copy cursor 2", "move right", "move left", "shrink", "broaden", "skew up", "skew down", "-write plot scale", "zoom X", "change cen&win", "zoom to all data"]
        n215 = Unbundle By Name(w545) -> ("window"=w549:dbl, "window"=w548:dbl, "default window frac"=w546:dbl)
        n216 = Multiply(x=w548, y=w546) -> (x*y=w547:dbl)
        n217 = Add(x=w549, y=w547) -> (x+y=w550:dbl)
        n218 = Bundle By Name(cluster=w545, "window"=w550) -> (w544:T1)
        n219 = call "cursor window action stack.vi"("stack action"=stack_action_--_control."push", "action list"=w551, "command stack"=w555) -> ("command stack out"=w554:T2[])  [unwired: 6 in, 2 out]
      }
      frame "skew up" {
        n220 = Unbundle By Name(w558) -> ("kind"=w557:enum16{"symmetric", "skewed", "fancy"})
        n221 = case shown="\"skewed\"" w557 {
          tunnel: w563 -> [w565 w575]
          tunnel: [w565 w574] -> w562
          tunnel: [w564 w573] -> w561
          tunnel: w558 -> [w564 w571]
          frame "symmetric", Default {
          }
          frame "skewed" {
            w577 = T2[] [enum."-change skew", enum."-read plot scale", enum."-set center.Y", enum."-write right.X", enum."-write left.X", enum."-write center.Y"] items=["balance", "h. offset change", "cursor moves", "change center", "change window", "init", "check", "reset", "set y to middle", "idle", "-write all Y", "-write left.X", "-write center.X", "-write right.X", "-write all X", "-change center", "-change window", "-change skew", "-read cursor 2", "-read cursor 1", "-read cursor 0", "-read all cursors", "-reset", "-read plot scale", "-set y to middle", "-Q: center.Y is visible", "-Q: window is visible", "-parse center.Y", "-right left from center", "-left move", "-right move", "-set center.Y", "-empty", "-set cursors to default", "-check", "-write center.Y", "-copy cursor 1", "-copy cursor 0", "-copy cursor 2", "move right", "move left", "shrink", "broaden", "skew up", "skew down", "-write plot scale", "zoom X", "change cen&win", "zoom to all data"]
            n222 = Unbundle By Name(w571) -> ("skew"=w572:dbl)
            n223 = Add(x=0.1, y=w572) -> (x+y=w569:dbl)
            n224 = call "Q -- check range -- i -- real.vi"("upper"=1, "lower"=-1, "number"=w569) -> ("number in range"=w566:dbl)  [unwired: 6 in, 2 out]
            n225 = Bundle By Name(cluster=w571, "skew"=w566) -> (w573:T1)
            n226 = call "cursor window action stack.vi"("stack action"=stack_action_--_control."push", "action list"=w577, "command stack"=w575) -> ("command stack out"=w574:T2[])  [unwired: 6 in, 2 out]
          }
        }
      }
      frame "skew down" {
        n227 = Unbundle By Name(w579) -> ("kind"=w578:enum16{"symmetric", "skewed", "fancy"})
        n228 = case shown="\"skewed\"" w578 {
          tunnel: w584 -> [w586 w597]
          tunnel: [w586 w596] -> w583
          tunnel: [w585 w595] -> w582
          tunnel: w579 -> [w585 w594]
          frame "symmetric", Default {
          }
          frame "skewed" {
            w589 = T2[] [enum."-change skew", enum."-read plot scale", enum."-set center.Y", enum."-write right.X", enum."-write left.X", enum."-write center.Y"] items=["balance", "h. offset change", "cursor moves", "change center", "change window", "init", "check", "reset", "set y to middle", "idle", "-write all Y", "-write left.X", "-write center.X", "-write right.X", "-write all X", "-change center", "-change window", "-change skew", "-read cursor 2", "-read cursor 1", "-read cursor 0", "-read all cursors", "-reset", "-read plot scale", "-set y to middle", "-Q: center.Y is visible", "-Q: window is visible", "-parse center.Y", "-right left from center", "-left move", "-right move", "-set center.Y", "-empty", "-set cursors to default", "-check", "-write center.Y", "-copy cursor 1", "-copy cursor 0", "-copy cursor 2", "move right", "move left", "shrink", "broaden", "skew up", "skew down", "-write plot scale", "zoom X", "change cen&win", "zoom to all data"]
            n229 = Unbundle By Name(w594) -> ("skew"=w588:dbl)
            n230 = Subtract(x=w588, y=0.1) -> (x-y=w593:dbl)
            n231 = call "Q -- check range -- i -- real.vi"("upper"=1, "lower"=-1, "number"=w593) -> ("number in range"=w590:dbl)  [unwired: 6 in, 2 out]
            n232 = Bundle By Name(cluster=w594, "skew"=w590) -> (w595:T1)
            n233 = call "cursor window action stack.vi"("stack action"=stack_action_--_control."push", "action list"=w589, "command stack"=w597) -> ("command stack out"=w596:T2[])  [unwired: 6 in, 2 out]
          }
        }
      }
      frame "-parse center.Y" {
        w611 = 1.0  # y
        w613 = 2.0  # y
        # "left factor"
        # "right factor"
        # "0 .. 1"
        # "-1 .. 1"
        # "-1..1"
        # "\"zero\""
        # "calculate horizontal offset and/or window \nfrom vertical position of center cursor"
        n234 = Unbundle By Name(w622) -> ("center.Y"=w607:dbl, "scale.y.max"=w605:dbl, "scale.y.min"=w606:dbl, "scale.y.center"=w603:dbl, "scale.y.halfwidth"=w615:dbl)
        n235 = Unbundle By Name(w618) -> ("fixed vertical offset"=w635:dbl)
        n236 = Multiply(x=w615, y=w635) -> (x*y=w633:dbl)
        n237 = call "Q -- check range -- i -- real.vi"("upper"=w605, "lower"=w606, "default"=w603, "number"=w607) -> ("number in range"=w604:dbl)  [unwired: 5 in, 2 out]
        n238 = Add(x=w633, y=w603) -> (x+y=w630:dbl)
        n239 = Unbundle By Name(w618) -> ("default window frac"=w623:dbl, "kind"=w624:enum16{"symmetric", "skewed", "fancy"}, "skew"=w620:dbl, "window"=w619:dbl)
        n240 = Unbundle By Name(w622) -> ("scale.x.range"=w621:dbl)
        n241 = Subtract(x=w630, y=w606) -> (x-y=w631:dbl)
        n242 = Subtract(x=w605, y=w630) -> (x-y=w632:dbl)
        n243 = Max & Min(x=w632, y=w631) -> (min(x,y)=w628:dbl)  [unwired: 1 out]
        n244 = Subtract(x=w604, y=w630) -> (x-y=w629:dbl)
        n245 = Divide(x=w629, y=w628) -> (x/y=w627:dbl)
        n246 = Multiply(x=w627, y=0.99) -> (x*y=w602:dbl)
        n247 = call "Q -- check range -- i -- real.vi"("upper"=1, "lower"=-1, "number"=w602) -> ("number in range"=w599:dbl)  [unwired: 6 in, 2 out]
        n248 = Bundle By Name(cluster=w622, "center.Y"=w604) -> (w625:T5)
        n249 = case shown="\"symmetric\", Default" w624 {
          tunnel: [w636 w647] -> w610
          tunnel: w599 -> [w645 w647]
          tunnel: w623 -> [w644 _]
          tunnel: w621 -> [w643 _]
          tunnel: [w637 w646] -> w617
          tunnel: w620 -> [w636 _]
          tunnel: w619 -> [_ w646]
          frame "symmetric", Default {
            # "0 .. 1"
            # "-1 .. 1"
            n250 = Add(x=w645, y=1.0) -> (x+y=w641:dbl)
            n251 = Divide(x=w641, y=2.0) -> (x/y=w639:dbl)
            n252 = Multiply(x=w644, y=w639) -> (x*y=w638:dbl)
            n253 = Multiply(x=w638, y=w643) -> (x*y=w637:dbl)
          }
          frame "skewed" {
          }
        }
        n254 = Add(x=w610, y=w611) -> (x+y=w612:dbl)
        n255 = Divide(x=w612, y=w613) -> (x/y=w608:dbl)
        n256 = Subtract(x=w611, y=w608) -> (x-y=w609:dbl)
        n257 = Bundle By Name(cluster=w618, "skew"=w610, "window"=w617, "skew.left"=w609, "skew.right"=w608) -> (w614:T1)
      }
      frame "-Q: window is visible" {
        n258 = Unbundle By Name(w658) -> ("scale.x.min"=w650:dbl, "scale.x.max"=w649:dbl, "scale.x.center"=w653:dbl, "scale.x.range"=w648:dbl)  [unwired: 1 out]
        n259 = Unbundle By Name(w652) -> ("center"=w657:dbl)
        n260 = call "Q -- check range -- i -- real.vi"("upper"=w649, "lower"=w650, "number"=w657) -> ("selector"=w656:T7)  [unwired: 6 in, 2 out]
        n261 = case shown="\"in range\"" w656 {
          tunnel: w655 -> [w665 w690]
          tunnel: [w664 w688] -> w654
          tunnel: w652 -> [w663 w687]
          tunnel: w653 -> [_ w686]
          tunnel: [w661 w685] -> w651
          tunnel: w650 -> [w671 _]
          tunnel: w649 -> [w670 _]
          tunnel: w648 -> [w662 _]
          frame "in range" {
            n262 = Unbundle By Name(w663) -> ("left"=w673:dbl, "right"=w672:dbl)
            n263 = call "Q -- check range -- i -- real.vi"("upper"=w670, "lower"=w671, "number"=w673) -> ("in range?"=w669:bool)  [unwired: 6 in, 2 out]
            n264 = call "Q -- check range -- i -- real.vi"("upper"=w670, "lower"=w671, "number"=w672) -> ("in range?"=w668:bool)  [unwired: 6 in, 2 out]
            n265 = Not(x=w669) -> (.not. x?=w667:bool)
            n266 = Not(x=w668) -> (.not. x?=w666:bool)
            n267 = And(x=w667, y=w666) -> (x .and. y?=w660:bool)
            n268 = case shown="True" w660 {
              tunnel: w665 -> [w675 w682]
              tunnel: [w675 w681] -> w664
              tunnel: w663 -> [w674 w680]
              tunnel: w662 -> [_ w678]
              tunnel: [w674 w676] -> w661
              frame False {
              }
              frame True {
                w684 = T2[] [enum."-change window", enum."-write left.X", enum."-write right.X"] items=["balance", "h. offset change", "cursor moves", "change center", "change window", "init", "check", "reset", "set y to middle", "idle", "-write all Y", "-write left.X", "-write center.X", "-write right.X", "-write all X", "-change center", "-change window", "-change skew", "-read cursor 2", "-read cursor 1", "-read cursor 0", "-read all cursors", "-reset", "-read plot scale", "-set y to middle", "-Q: center.Y is visible", "-Q: window is visible", "-parse center.Y", "-right left from center", "-left move", "-right move", "-set center.Y", "-empty", "-set cursors to default", "-check", "-write center.Y", "-copy cursor 1", "-copy cursor 0", "-copy cursor 2", "move right", "move left", "shrink", "broaden", "skew up", "skew down", "-write plot scale", "zoom X", "change cen&win", "zoom to all data"]
                n269 = Unbundle By Name(w680) -> ("default window frac"=w679:dbl)
                n270 = Multiply(x=w679, y=w678) -> (x*y=w677:dbl)
                n271 = Bundle By Name(cluster=w680, "window"=w677) -> (w676:T1)
                n272 = call "cursor window action stack.vi"("stack action"=stack_action_--_control."push", "action list"=w684, "command stack"=w682) -> ("command stack out"=w681:T2[])  [unwired: 6 in, 2 out]
              }
            }
          }
          frame "not a number", "above", "below", Default {
            w691 = T2[] [enum."-change center", enum."-write all X", enum."-Q: window is visible"] items=["balance", "h. offset change", "cursor moves", "change center", "change window", "init", "check", "reset", "set y to middle", "idle", "-write all Y", "-write left.X", "-write center.X", "-write right.X", "-write all X", "-change center", "-change window", "-change skew", "-read cursor 2", "-read cursor 1", "-read cursor 0", "-read all cursors", "-reset", "-read plot scale", "-set y to middle", "-Q: center.Y is visible", "-Q: window is visible", "-parse center.Y", "-right left from center", "-left move", "-right move", "-set center.Y", "-empty", "-set cursors to default", "-check", "-write center.Y", "-copy cursor 1", "-copy cursor 0", "-copy cursor 2", "move right", "move left", "shrink", "broaden", "skew up", "skew down", "-write plot scale", "zoom X", "change cen&win", "zoom to all data"]
            n273 = Bundle By Name(cluster=w687, "center"=w686) -> (w685:T1)
            n274 = call "cursor window action stack.vi"("stack action"=stack_action_--_control."push", "action list"=w691, "command stack"=w690) -> ("command stack out"=w688:T2[])  [unwired: 6 in, 2 out]
          }
        }
      }
      frame "-write all X" {
        w708 = enum16{"", "read", "write"}."write"  # action
        n275 = Unbundle By Name(w692) -> ("Plot ref"=w693:refnum<vi>, "cursors"=w706:i32[], "left"=w700:dbl, "center"=w699:dbl, "right"=w698:dbl)
        n276 = Index Array(array=w706, index #1=0 ("cursor index"), index #2=1 ("cursor index"), index #3=2 ("cursor index")) -> (element #1=w707:i32, element #2=w703:i32, element #3=w701:i32)
        n277 = call "replace cursor - plot ref.vi"("action"=w708, "cursor index"=w707, "new X"=w700, "Plot ref in"=w693) -> ("Plot ref out"=w697:refnum<vi>)  [unwired: 5 in, 2 out]
        n278 = call "replace cursor - plot ref.vi"("action"=w708, "cursor index"=w703, "new X"=w699, "Plot ref in"=w697) -> ("Plot ref out"=w696:refnum<vi>)  [unwired: 5 in, 2 out]
        n279 = call "replace cursor - plot ref.vi"("action"=w708, "cursor index"=w701, "new X"=w698, "Plot ref in"=w696) -> ()  [unwired: 5 in, 3 out]
      }
      frame "-write all Y" {
        w726 = enum16{"", "read", "write"}."write"  # action
        n280 = Unbundle By Name(w714) -> ("Plot ref"=w715:refnum<vi>, "cursors"=w724:i32[])
        n281 = Unbundle By Name(w713) -> ("left.Y"=w712:dbl, "center.Y"=w711:dbl, "right.Y"=w710:dbl)
        n282 = Index Array(array=w724, index #1=0 ("cursor index"), index #2=1 ("cursor index"), index #3=2 ("cursor index")) -> (element #1=w725:i32, element #2=w721:i32, element #3=w719:i32)
        n283 = call "replace cursor - plot ref.vi"("action"=w726, "cursor index"=w725, "new  Y"=w712, "Plot ref in"=w715) -> ("Plot ref out"=w718:refnum<vi>)  [unwired: 5 in, 2 out]
        n284 = call "replace cursor - plot ref.vi"("action"=w726, "cursor index"=w721, "new  Y"=w711, "Plot ref in"=w718) -> ("Plot ref out"=w717:refnum<vi>)  [unwired: 5 in, 2 out]
        n285 = call "replace cursor - plot ref.vi"("action"=w726, "cursor index"=w719, "new  Y"=w710, "Plot ref in"=w717) -> ()  [unwired: 5 in, 3 out]
      }
      frame "-write left.X" {
        w741 = enum16{"", "read", "write"}."write"  # action
        n286 = Unbundle By Name(w728) -> ("Plot ref"=w733:refnum<vi>, "cursors"=w739:i32[], "left"=w729:dbl, "right"=w730:dbl, "wing order"=w732:enum16{"forw", "back"})
        n287 = Index Array(array=w739, index #1=0 ("cursor index"), index #2=1 ("cursor index"), index #3=2 ("cursor index")) -> (element #1=w740:i32)  [unwired: 2 out]
        n288 = case shown="\"back\"" w732 {
          tunnel: [w743 w744] -> w731
          tunnel: w730 -> [_ w744]
          tunnel: w729 -> [w743 _]
          frame "forw", Default {
          }
          frame "back" {
          }
        }
        n289 = call "replace cursor - plot ref.vi"("action"=w741, "cursor index"=w740, "new X"=w731, "Plot ref in"=w733) -> ()  [unwired: 5 in, 3 out]
      }
      frame "-write right.X" {
        w758 = enum16{"", "read", "write"}."write"  # action
        n290 = Unbundle By Name(w745) -> ("Plot ref"=w751:refnum<vi>, "cursors"=w757:i32[], "left"=w747:dbl, "right"=w748:dbl, "wing order"=w750:enum16{"forw", "back"})
        n291 = Index Array(array=w757, index #1=0 ("cursor index"), index #2=1 ("cursor index"), index #3=2 ("cursor index")) -> (element #3=w746:i32)  [unwired: 2 out]
        n292 = case shown="\"back\"" w750 {
          tunnel: [w760 w761] -> w749
          tunnel: w748 -> [w760 _]
          tunnel: w747 -> [_ w761]
          frame "forw", Default {
          }
          frame "back" {
          }
        }
        n293 = call "replace cursor - plot ref.vi"("action"=w758, "cursor index"=w746, "new X"=w749, "Plot ref in"=w751) -> ()  [unwired: 5 in, 3 out]
      }
      frame "-write center.X" {
        w772 = enum16{"", "read", "write"}."write"  # action
        n294 = Unbundle By Name(w764) -> ("Plot ref"=w765:refnum<vi>, "cursors"=w771:i32[], "center"=w762:dbl)
        n295 = Index Array(array=w771, index #1=0 ("cursor index"), index #2=1 ("cursor index"), index #3=2 ("cursor index")) -> (element #2=w763:i32)  [unwired: 2 out]
        n296 = call "replace cursor - plot ref.vi"("action"=w772, "cursor index"=w763, "new X"=w762, "Plot ref in"=w765) -> ()  [unwired: 5 in, 3 out]
      }
      frame "-write center.Y" {
        w784 = enum16{"", "read", "write"}."write"  # action
        n297 = Unbundle By Name(w777) -> ("Plot ref"=w778:refnum<vi>, "cursors"=w783:i32[])
        n298 = Index Array(array=w783, index #1=0 ("cursor index"), index #2=1 ("cursor index"), index #3=2 ("cursor index")) -> (element #2=w774:i32)  [unwired: 2 out]
        n299 = Unbundle By Name(w776) -> ("center.Y"=w775:dbl)
        n300 = call "replace cursor - plot ref.vi"("action"=w784, "cursor index"=w774, "new  Y"=w775, "Plot ref in"=w778) -> ()  [unwired: 5 in, 3 out]
      }
      frame "-read all cursors" {
        w806 = enum16{"", "read", "write"}."read"  # action
        n301 = Unbundle By Name(w786) -> ("Plot ref"=w787:refnum<vi>, "cursors"=w804:i32[])
        n302 = Index Array(array=w804, index #1=0 ("cursor index"), index #2=1 ("cursor index"), index #3=2 ("cursor index")) -> (element #1=w805:i32, element #2=w801:i32, element #3=w799:i32)
        n303 = call "replace cursor - plot ref.vi"("action"=w806, "cursor index"=w805, "Plot ref in"=w787) -> ("read Y"=w793:dbl, "read X"=w794:dbl, "Plot ref out"=w798:refnum<vi>)  [unwired: 6 in]
        n304 = call "replace cursor - plot ref.vi"("action"=w806, "cursor index"=w801, "Plot ref in"=w798) -> ("read Y"=w791:dbl, "read X"=w792:dbl, "Plot ref out"=w797:refnum<vi>)  [unwired: 6 in]
        n305 = call "replace cursor - plot ref.vi"("action"=w806, "cursor index"=w799, "Plot ref in"=w797) -> ("read Y"=w789:dbl, "read X"=w790:dbl)  [unwired: 6 in, 1 out]
        n306 = Bundle By Name(cluster=w796, "left.X"=w794, "left.Y"=w793, "center.X"=w792, "center.Y"=w791, "right.X"=w790, "right.Y"=w789) -> (w795:T5)
      }
      frame "-read cursor 2" {
        w820 = enum16{"", "read", "write"}."read"  # action
        n307 = Unbundle By Name(w809) -> ("Plot ref"=w810:refnum<vi>, "cursors"=w819:i32[])
        n308 = Index Array(array=w819, index #1=0 ("cursor index"), index #2=1 ("cursor index"), index #3=2 ("cursor index")) -> (element #3=w808:i32)  [unwired: 2 out]
        n309 = call "replace cursor - plot ref.vi"("action"=w820, "cursor index"=w808, "Plot ref in"=w810) -> ("read Y"=w812:dbl, "read X"=w813:dbl)  [unwired: 6 in, 1 out]
        n310 = Bundle By Name(cluster=w815, "right.X"=w813, "right.Y"=w812) -> (w814:T5)
      }
      frame "-read cursor 1" {
        w834 = enum16{"", "read", "write"}."read"  # action
        n311 = Unbundle By Name(w822) -> ("Plot ref"=w824:refnum<vi>, "cursors"=w833:i32[])
        n312 = Index Array(array=w833, index #1=0 ("cursor index"), index #2=1 ("cursor index"), index #3=2 ("cursor index")) -> (element #2=w823:i32)  [unwired: 2 out]
        n313 = call "replace cursor - plot ref.vi"("action"=w834, "cursor index"=w823, "Plot ref in"=w824) -> ("read Y"=w826:dbl, "read X"=w827:dbl)  [unwired: 6 in, 1 out]
        n314 = Bundle By Name(cluster=w829, "center.X"=w827, "center.Y"=w826) -> (w828:T5)
      }
      frame "-read cursor 0" {
        w848 = enum16{"", "read", "write"}."read"  # action
        n315 = Unbundle By Name(w836) -> ("Plot ref"=w838:refnum<vi>, "cursors"=w847:i32[])
        n316 = Index Array(array=w847, index #1=0 ("cursor index"), index #2=1 ("cursor index"), index #3=2 ("cursor index")) -> (element #1=w837:i32)  [unwired: 2 out]
        n317 = call "replace cursor - plot ref.vi"("action"=w848, "cursor index"=w837, "Plot ref in"=w838) -> ("read Y"=w840:dbl, "read X"=w841:dbl)  [unwired: 6 in, 1 out]
        n318 = Bundle By Name(cluster=w843, "left.X"=w841, "left.Y"=w840) -> (w842:T5)
      }
    }
    n319 = call "cursor window action stack.vi"("stack action"=stack_action_--_control."check", "command stack"=w28) -> ("stack is empty ?"=w26:bool, "command stack out"=w27:T2[])  [unwired: 7 in, 1 out]
  }
  "cursor window out" <- w10
  n320 = property class="Clust (strict)"(reference=w19, "Value"=w10) -> (reference out=→"cursor window out":refnum<vi>)  [unwired: 1 in, 1 out]
